vi "UHR-Fleezers Control (fpga) - Leonardo 04-2018 V3.vi"() -> ()   [LabVIEW 2013]
doc: "UHR-Fleezers Instrument Control Code (fpga)"
uses:
  <vilib>/Platform/TimedLoop/XDataNode/timing_clust.ctl
  <vilib>/Platform/TimedLoop/XDataNode/nitl_modes.ctl
  <vilib>/Platform/TimedLoop/XDataNode/wakeup.ctl
  <vilib>/rvi/eio/common/nirviEmuTemplateMethod_errors.vi
  <vilib>/rvi/Emulation/niFpgaSctlEmulationGetInTimedLoop.vi
  <vilib>/rvi/Emulation/niFpgaEmulationReportErrorSimple.vi
  <vilib>/rvi/Emulation/niFpgaGetClockAttributes.vi
  <vilib>/rvi/Emulation/niFpgaCriticalErrorInLSC.vi
  <vilib>/rvi/FIFO/Fifo_Resource/nirvififoEmulationReadFpgaImpl.vi
  <vilib>/rvi/DataTransferAndStorage/Container/Common/niFpgaContainerGetUniqueNameForEmu.vi
  <vilib>/rvi/DataTransferAndStorage/Container/Common/niFpgaContainerExecOnDevCompGetState.vi
  <vilib>/rvi/interface/RandomDataEmulation/nirviRandomDataFPGAFIFO.vi
  <vilib>/rvi/interface/RandomDataEmulation/niFpgaRandomDataHandleErrors.vi
  <vilib>/rvi/eio/common/nirviEmuReportErrorAndStop.vi
  <vilib>/rvi/Emulation/niFpgaProcessEmulError.vi
  <vilib>/rvi/FIFO/Fifo_Resource/nirvififoEmulationWriteFpgaImpl.vi
  <vilib>/Platform/TimedLoop/XDataNode/XDataNode.xnode
  <vilib>/eio/EIOMethodNode/EIOMethodNode.xnode
  <vilib>/eio/EIONode/EIONode.xnode
  <vilib>/rvi/DataTransferAndStorage/Container/XNode/niFpgaContainer.xnode
  <vilib>/rvi/FIFO/Fifo_Resource/nirvififoEmulationRead.vi
  <vilib>/rvi/FIFO/Fifo_Resource/niFpgaFifoEmulationRefIn.vi
  <vilib>/rvi/interface/RandomDataEmulation/nirviRandomDataFpgaReadWriteTemplate.vi
  <vilib>/rvi/FIFO/Fifo_Resource/nirvififoEmulationWrite.vi
  <vilib>/addons/control/pid/fpga.llb/XNode/niFpgaPID.xnode
  <vilib>/Platform/TimedLoop/XDataNode/XDNodeRunTimeDep.lvlib
  <vilib>/rvi/Memory/Memory_Emulation/niFpgaMemoryEmulationRefIn.vi
panel:
  in  "Tab Control 2":T1(tab)
  out "BD1 amplitude 1 out":u16
  out "BD1 amplitude 2 out":u16
  in  "FB output range":cluster{"output low":i16, "output high":i16}={"output low"=0, "output high"=3000}
  in  "FB Gains":T2={"proportional gain (Kc)"=10, "integral gain (Kc*Ts/Ti)"=5, "derivative gain (Kc*Td/Ts)"=0}
  in  "RF synth green feedback max":i16=4000
  in  "RD":bool=TRUE
  in  "Swap F1 and F2":bool
  in  "Scan BD":bool
  in  "Start scan":bool
  in  "OSK Bd 1":bool
  in  "Reset Bd 1":bool
  in  "PMODE":bool=TRUE
  in  "Number Interlace Cycles":u8=2 min=1 max=3
  in  "Interlace Off Parameters":u8=1 min=1 max=3
  in  "Interlace ON/OFF":bool
  out "DIO Relative phase":i16
  in  "Phase count adjustment (DIO)":i16
  in  "+ phase (DIO)":bool
  out "DIO Late Counter":u8
  in  "DIO count 1 (ticks)":u16=400
  in  "DIO count 2 (ticks)":u16=400
  in  "DIO count 3 (ticks)":u16=400
  out "AI2 Y Sum Set 2":i16
  out "AI2 Y Sum Set 1":i16
  in  "FB Setpoint Set 1":i16 min=0 step=1
  in  "FB Reset Set 1":bool
  in  "FB On/Off Set 1":bool
  in  "FB Reset Set 2":bool
  in  "FB On/Off Set 2":bool
  in  "FB Setpoint Set 2":i16 min=0 step=1
  in  "Amp switch delay":u8=5
  in  "RF synth bd controls green":bool
  in  "Phase Trap 2":fxp<+,14,14>
  in  "Phase Trap 1":fxp<+,14,14>
  in  "Phase offset method":u8
  in  "BD 2 Amplitude 1":u16
  in  "BD 1 Amplitude 1":u16
  in  "BD 2 Frequency 1":u64
  in  "BD 1 Frequency 1":u64
  in  "BD 2 Amplitude 2":u16
  in  "BD 1 Amplitude 2":u16
  in  "BD 2 Frequency 2":u64
  in  "BD 1 Frequency 2":u64
  in  "BD 2 Amplitude 3":u16
  in  "BD 1 Amplitude 3":u16
  in  "BD 2 Frequency 3":u64
  in  "BD 1 Frequency 3":u64
  in  "BD 2 Delay (Ticks)":u8 caption="Count(Ticks)"
  in  "Next trap write delay (ticks)":u8 caption="Count(Ticks)"
  out "Random phase generated":fxp<+,14,14>
  in  "RF phase reset before cycles":bool
  in  "Trap 1 osc enable":bool
  in  "N trap osc periods":i16
  in  "Trap osc period (pts)":i16
  in  "Osc traps":bool
  in  "Initiate trap osc":bool
  in  "Ready Write":bool
  in  "Data":i64
  in  "Address 2":u32
  in  "Osc trap cont.":bool
  in  "Trap 2 osc enable":bool
  out "green FB running":bool
  in  "APD 2 AO scale factor":i16=1
  in  "BD 1 Delay (ticks)":u8
  in  "Tab Control":T3(tab)=enum."MCL trap control"
  in  "Set 3":bool
  in  "Set 2":bool=TRUE
  in  "Set 1":bool=TRUE
  in  "Trap Pos to FIFO":bool
  in  "N of AI1 Int Acq Sets":i16=2 min=1 max=3 step=1
  out "AI Late Counter":u8
  in  "ai count":u16=400
  in  "+ phase":bool
  in  "Phase count adjustment":i16
  out "Relative phase":i16
  in  "AI to FIFO":bool
  out "BD1 Frequency Out 1":u64
  out "BD1 Frequency Out 2":u64
  out "Trap Pos FIFO Timeout":u16
  out "Trap AI FIFO Timeout":u16
  in  "Trap FIFO Set Timeout":i32
  in  "Scan freq.  increment":i64
  in  "Scan steps":u64
  in  "Number of scans":u16
  in  "Cycles per step":u64
  in  "Raster setpoint":fxp<+/-,16,1>
  in  "Raster to target force":bool
  out "Actual Scan freq":u64
  in  "Cont. Scan":bool
  out "Scan I":u64
  in  "Abort scan":bool
  out "Scanning":bool
  in  "FB Min frequency":u64
  in  "FB Max Frequency":u64
  in  "Dynamic Force FB (Ronen)":bool
  in  "Trap pos. FB Range":T4={"FB2 output low"=-1.0, "FB2 output high"=0.999969482421875}
  in  "Trap Pos. FB Gains":T5={"proportional gain (Kc)"=0.999969482421875, "integral gain (Kc*Ts/Ti)"=0.999969482421875, "derivative gain (Kc*Td/Ts)"=0.0}
  in  "B factor":fxp<+/-,32,16>
  in  "Negate Diff?":bool
  in  "Diff FB Measurement?":bool
  in  "FB Trig Integrate":u32=1
  out "TTrig?":bool
  in  "TTrig Negate Pos":bool=TRUE
  out "Trap Pos FB Int Signal":fxp<+/-,24,9> format="%.18g"
  out "Trap Pos FB Int-Norm Signal":fxp<+/-,16,1> format="%.16g"
  in  "FPGA TTrig Thresh":i64
  in  "FPGA Trap Trig":bool
  out "Trap Pos FB Action":i64
  in  "Trap Pos. FB Offset Factor":i64
  in  "Trap Pos. FB Mult Factor":i64=2
  in  "Trap Pos. FB Reset":bool
  in  "Trap Pos FB Monitor T1 or T2":bool
  in  "AI1 X Scale":u16
  in  "Trap Pos FB Int Count":u16=100
  in  "Trap Pos FB Negate Action":bool
  out "AI1 X Set 2":fxp<+/-,16,1>
  out "AI1 X Set 1":fxp<+/-,16,1>
  in  "Trap Pos. FB SP":fxp<+/-,16,1>
  in  "Force feedback":bool
  out "TTrig Sig":i64
  out "TTrig Fin Thresh":i64
  in  "1D or 2D Scan?":bool
  in  "Abort scan (MCL)":bool
  in  "MCL Scan Axis":bool
  in  "Cont. Scan (MCL)":bool
  out "Scan I (MCL)":u64
  in  "Number of scans (MCL)":u16
  out "Scanning MCL":bool
  in  "Scan steps (MCL)":u64
  in  "Cycles per step (MCL)":u64
  in  "Scan freq.  increment (MCL)":i16
  in  "Start scan (MCL)":bool
  in  "AO2 (X)":i16
  in  "AO1 (Y)":i16
  out "MCL Late Counter":u8
  in  "MCL count":u32=800
  out "MCL Relative Phase":i16
  in  "Phase count adjustment (MCL)":i16
  in  "+ phase (MCL)":bool
  in  "Lifetime events to read blue":u16=100
  in  "Lifetime read blue fifo":bool
  out "lifetime events in fifo":u16
  in  "APD Gate Operating Mode":u8 max=2 step=1
  in  "Invert APD Gate":bool
  in  "APD Gate OFF Count":u16=100
  in  "APD Gate ON Count":u16=300
  out "APD 1 Gate Late Counter":u8
  out "APD 1 Gate Relative Phase":i16
  in  "Phase count adjustment (APD 1 Gate)":i16
  in  "+ phase (APD 1 Gate)":bool
  out "APD 2 Counts 0":u32
  out "APD 2 Counts 1":u32
  out "APD 1 Counts 0":u32
  out "APD 1 Counts 1":u32
  in  "Lifetime timeout APD1":u16=200
  in  "APD to FIFO":bool
  in  "APD Acq Rate Count":u32=20000000
  out "APD Acq Late Counter":u16
  out "APD Acq Relative Phase":i16
  in  "+ phase (APD Acq)":bool
  in  "Phase Count Adjustment (APD Acq)":i16
  in  "APD 1 AO scale factor":i16=1
  out "APD2 out state":bool
  out "APD1 out state":bool
  out "APD Acq Late?":bool
  in  "D3 2":i16
  in  "I3 2":i16=5
  in  "P3 2":i16=10
  in  "Green FB Setpoint 2":i16=250 min=0 step=1
  in  "Green FB Reset 2":bool
  in  "Green Filter Flipper":bool
  in  "Green interlace OFF count":u16=100
  out "GI Relative phase":i16
  in  "Phase count adjustment (GI)":i16
  in  "+ phase (GI)":bool
  in  "Green interlace ON count":u16=300
  out "GI Late Counter":u8
  in  "Invert GI":bool
  in  "Operating Mode":u8 max=2 step=1
  in  "Current Out":u16=30000
  in  "Green int current ON count adj":u32=150
  in  "Green interlace OFF count 2":u32=900
  in  "Green interlace ON count 2":u32=300
  out "GI Late Counter 2":u16
  in  "Green FB Count":u32=1200
  in  "Phase count adjustment (GI) 2":i16=20
  in  "Green FB Setpoint":i16=250 min=0 step=1
  in  "Invert GI 2":bool
  out "GI Relative phase 2":i16
  in  "+ phase (GI) 2":bool
  in  "Phase count adjustment (Green FB)":i16=10
  out "Green Late Counter":u16
  out "Green FB Relative Phase":i16
  in  "+ phase (Green FB)":bool
  out "Green FB Signals":T6
  out "Green FB Sum":i16
  in  "Green FB Gains":T2={"proportional gain (Kc)"=10, "integral gain (Kc*Ts/Ti)"=5, "derivative gain (Kc*Td/Ts)"=0}
  in  "Green FB On/Off":bool
  in  "Green FB Reset":bool
  out "Green FB Late?":bool
  out "GI Late?":bool
  in  "Operating Mode 2":u8=2 max=2 step=1
  in  "Chassis2/Mod4/AO1":u16
  in  "+ phase (RI)":bool
  out "RI Relative phase":i16
  out "RI Late Counter":u8
  in  "Red interlace ON count":u16=300
  in  "Red interlace OFF count":u16=100
  in  "Invert RI":bool
  in  "Red Laser Operating Mode":u8 max=2 step=1
  in  "Phase count adjustment (RI)":i16
  in  "Phase count adjustment (BI D)":i16
  in  "Blue Laser Operating Mode (D)":u8 max=2 step=1
  in  "Invert BI (D)":bool
  in  "Blue interlace OFF count (D)":u16=100
  in  "Blue interlace ON count (D)":u16=300
  out "Blue Late Counter (D)":u8
  out "BI Relative phase (D)":i16
  in  "+ phase (BI D)":bool
  in  "Lifetime to FIFO":bool
  out "lifetime (ticks)":u16
  # "Raster Scan AOD"
  # "1 (X)"
  # "2 (Y)"
  # "IR Intensity Feedback (RF BD 1)"
  # "FB Gains Set 1"
  # "FB output range 1"
  # "IR Intensity Feedback (RF BD 2) -\nonly when using BD 2 for green laser AOM (not trap Y)"
  # "Keep below 4096 (12 bits) to stay within range of RF board. Going over doesn't saturate, it truncates higher bits."
  # "RF phase offset control"
  # "Methods are:\n0 - Default, do nothing at all (no phase offset writes)\n1 - Manual phase adjustment\n2 - Cycle the phase adjustment using the input phase numbers as increment values for each cycle"
  # "False is usual, True is external loop method"
  # "Parameters if using the external RF switching loop"
  # "Parameters if using the usual internal RF switching method"
  # "FB Triggering Excitation Laser"
  # "Trap Pos. FB Gains"
  # "Trap Pos. FB Range"
  # "AO1 (Y)"
  # "2D"
  # "Trap 3"
  # "1D"
  # "AO2 (X)"
  # "Fl Laser"
  # "APD AO for aligning"
  # "Detection Loop"
  # "Green fluorescent laser digital gate interlacing loop"
  # "0 Forced ON\n1 Forced OFF\n2 Interlacing"
  # "ALEX settings:"
  # "Controls for usual IA ME controls green AOM"
  # "Controls for RF synth board controls green AOM"
  # "Green FB Gains"
  # "Red fluorescent laser digital gate interlacing loop"
  # "Detection Loop"
  # "0 Forced ON\n1 Forced OFF\n2 Interlacing"
  # "Analog/FB Control Loop\n(Disabled)"
  # "Digital Control Loop"
  # "Blue laser intensity reading"
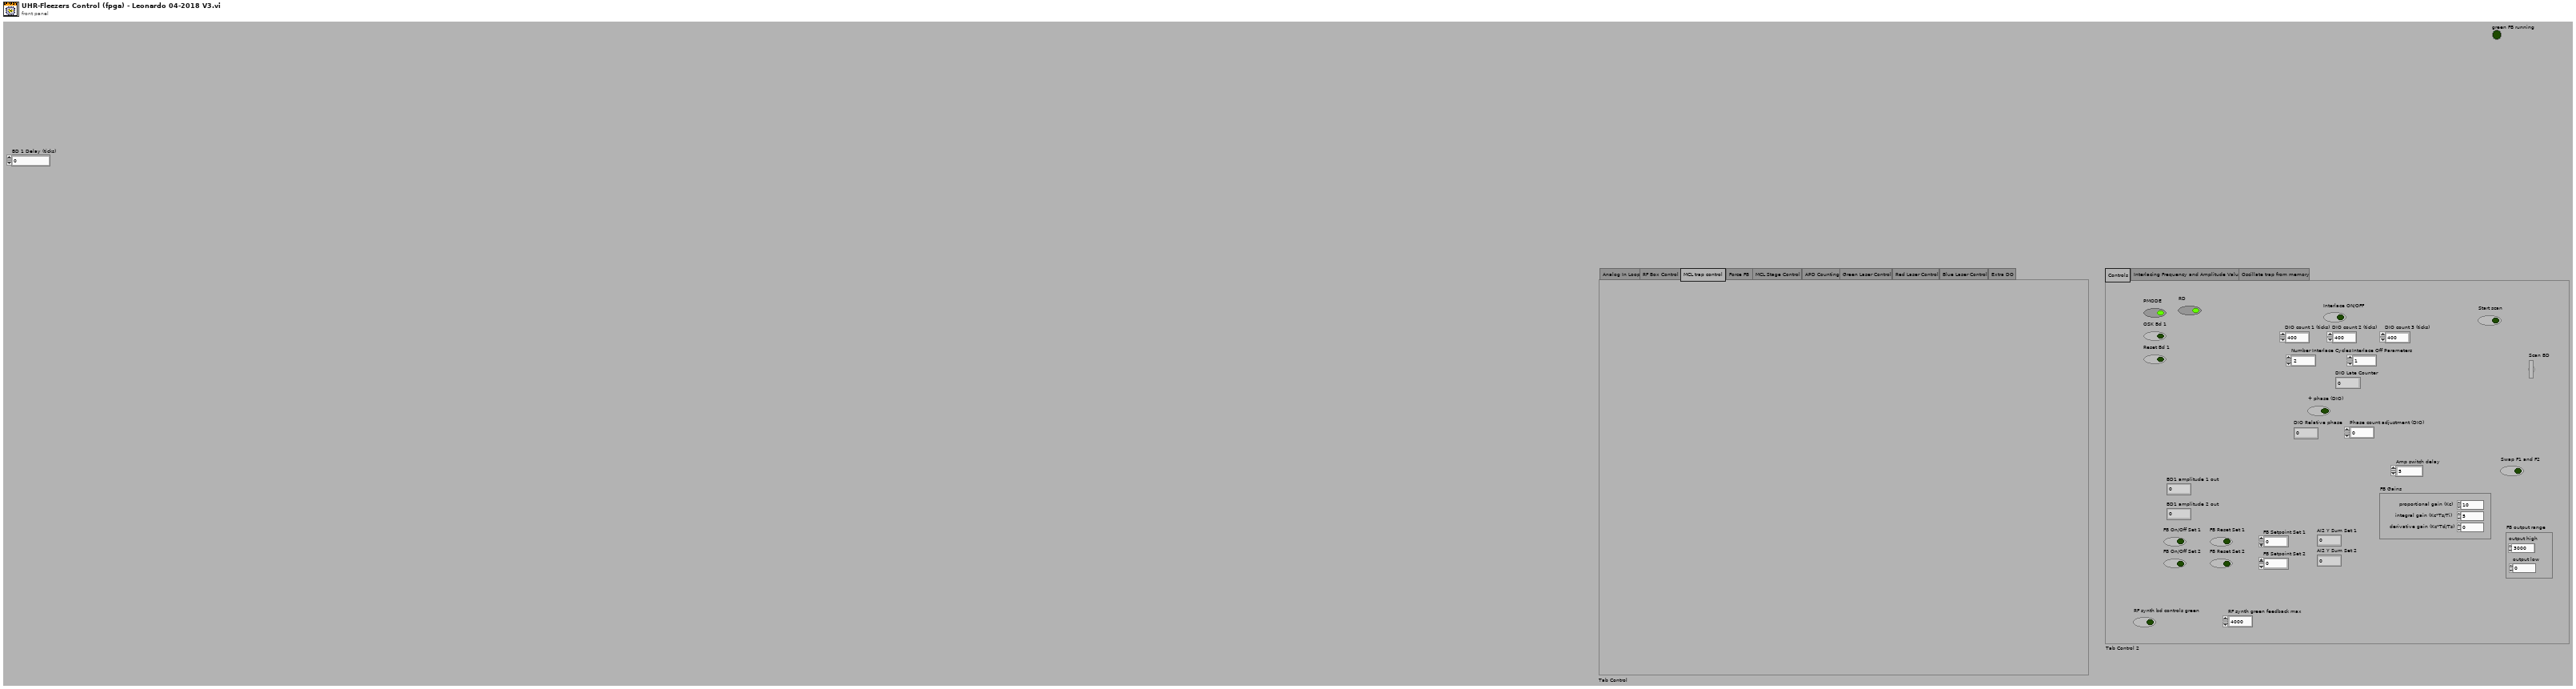
[diagram p1: front panel]
types:
  T1 = enum32{"Controls", "Interlacing Frequency and Amplitude Values", "Oscillate trap from memory"}
  T2 = cluster{"proportional gain (Kc)":i16, "integral gain (Kc*Ts/Ti)":i16, "derivative gain (Kc*Td/Ts)":i16}
  T3 = enum32{"Analog In Loop", "RF Box Control", "MCL trap control", "Force FB", "MCL Stage Control", "APD Counting", "Green Laser Control", "Red Laser Control", "Blue Laser Control", "Extra DO"}
  T4 = cluster{"FB2 output low":fxp<+/-,16,1>, "FB2 output high":fxp<+/-,16,1>}
  T5 = cluster{"proportional gain (Kc)":fxp<+/-,16,1>, "integral gain (Kc*Ts/Ti)":fxp<+/-,16,1>, "derivative gain (Kc*Td/Ts)":fxp<+/-,16,1>}
  T6 = cluster{"Green FB Ch 0":i16, "Green FB Ch 1":i16, "Green FB Ch 2":i16}
  T7 = typedef "XDNodeRunTimeDep.lvlib/timing_clust.ctl" = cluster{"Expected End [f-1]":u64, "Actual End [f-1]":u64, "Finished Late? [f-1]":bool, "Expected End [i-1]":u64, "Actual End [i-1]":u64, "Finished Late? [i-1]":bool, "Expected Start [i]":u64, "Actual Start [i]":u64, "Expected Start [f]":u64, "Actual Start [f]":u64, "Source Name":string, "Structure Name":string, "Period":i64, "Deadline":i64, "Offset":i64, "Start":i64, "Priority":i32, "Timeout":i32, "Mode":T8, "Wakeup Reason":T9, "Error":errorcluster, "Source Type":string, "Secondary Source Type":string, "Global End Time":u64, "Global Start Time":u64, "Frame Duration":u64, "Iteration Duration":u64, "Assigned CPU":i32, "I/O Scan Engine Mode":u32}
  T8 = typedef "XDNodeRunTimeDep.lvlib/nitl_modes.ctl" = enum32{"No Change", "Process missed periods, maintain original phase", "Discard missed periods, maintain original phase", "Process missed periods, ignore original phase", "Discard missed periods, ignore original phase"}
  T9 = typedef "XDNodeRunTimeDep.lvlib/wakeup.ctl" = enum32{"Normal", "Aborted", "Asynchronous wakeup", "Timing source error", "Timed loop error", "Timeout"}
  T10 = cluster{"Chassis2/Mod2/AI0":i16, "Chassis2/Mod2/AI1":i16, "Chassis2/Mod2/AI2":i16}
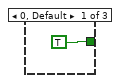
[diagram p3: hidden frame]
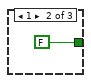
[diagram p4: hidden frame]
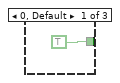
[diagram p8: hidden frame]
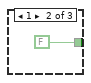
[diagram p9: hidden frame]
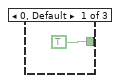
[diagram p10: hidden frame]
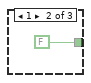
[diagram p11: hidden frame]
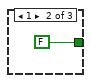
[diagram p13: hidden frame]
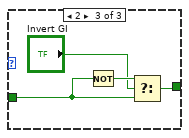
[diagram p14: hidden frame]
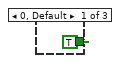
[diagram p15: hidden frame]
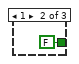
[diagram p16: hidden frame]
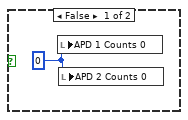
[diagram p17: hidden frame]
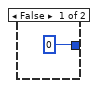
[diagram p19: hidden frame]
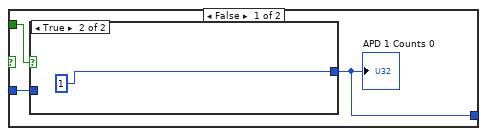
[diagram p20: hidden frame]
diagram:
  w5 = FALSE
  # "BD2 amp"
  # "BD1 amp"
  # "BD2 amp"
  # "BD1 amp"
  # "timing array current index"
  # "timing array"
  # "timing counter (phase adjusted here)"
  # "late counter"
  n1 = while {
    stop <- FALSE stop-if-true
    n2 = xnode "FPGA I/O Node"("Connector0/DIO3"="Green Filter Flipper", "Chassis2/Mod1/AO1"="Chassis2/Mod4/AO1") -> ()  [unwired: 2 in, 2 out]
    n3 = call "Loop Timer11"("Count(Ticks)"=u32 40000 ("Extra DO Counts")) -> ()  [unwired: 1 out]
  }
  n4 = disable-structure shown="Disabled" {
    frame Disabled {
      w20 = i16 2 items=["UnSet Ready", "ReadWrite", "Wait Ready"]
      n5 = while "Handshake memory transfer for trap oscillation sin wave data" {
        shift-right: [w22] -> _
        shift-left: w20 -> [w23]
        stop <- FALSE stop-if-true
        # "Write"
        n6 = case shown="1" w23 {
          tunnel: [w26 w31 w32] -> w22
          frame 3, Default {
            w24 = i16 2 items=["UnSet Ready", "ReadWrite", "Wait Ready"]
            w25 = i16 1 items=["UnSet Ready", "ReadWrite", "Wait Ready"]
            n7 = Select(t=w25, s="Ready Write", f=w24) -> (s? t:f=w26:i16)
          }
          frame 1 {
            w31 = i16 0 items=["UnSet Ready", "ReadWrite", "Wait Ready"]
            n8 = xnode ("Memory Write")("Address"="Address 2", "Data"="Data", "Memory In"=refnum<k21> "Trap osc memory") -> ()  [unwired: 1 out]
          }
          frame 0 {
            w32 = i16 2 items=["UnSet Ready", "ReadWrite", "Wait Ready"]
            n9 = local write "Ready Write"(FALSE ("Ready Read")) -> ()
          }
        }
      }
    }
    frame Enabled {
    }
  }
  n10 = flat-sequence "FPGA initialization to do before running any of the loops" {
    tunnel: [u16 0 ("DIO count 3 (ticks)")] -> w2
    tunnel: [w41] -> _
    frame #0 {
      # "UDCLK out enable and set low"
      # "WR"
      # "BD 2"
      # "BD 1"
      # "With the RF synth board initialization now done in a separate fpga vi, now when this vi is started, board is already configured and is ready for interlacing. Just need to set WR high and enabled UDCLK as write and set to low.\nbefore setting data and address bits."
      # "Start up expansion chassis early\nto avoid delays later"
      # "Set data and address values to something safe (a correct setting) so any initial WR and udclk flipping doesn't have a chance to mess anything up. Safe would be setting an unused data entry:"
      n11 = xnode "FPGA I/O Method Node"("Enable"=TRUE) -> ("FPGA I/O Out"=w35:refnum<k21>)  [unwired: 1 in]
      n12 = xnode "FPGA I/O Method Node"("Enable"=TRUE) -> ("FPGA I/O Out"=w38:refnum<k21>)  [unwired: 1 in]
      n13 = xnode "FPGA I/O Node"("Chassis2/Mod1/AO0"=u16 0 ("Chassis2/Mod4/AO0")) -> ("Chassis2/Mod2/AI0"=w41:i16)  [unwired: 2 in, 2 out]
      n14 = xnode "FPGA I/O Node"("Connector1/DIO15"=TRUE) -> ()  [unwired: 1 in, 1 out]
      n15 = xnode "FPGA I/O Node"("I/O Item"=FALSE ("Connector1/DIO30"), "FPGA I/O In"=w35) -> ()  [unwired: 1 out]
      n16 = xnode "FPGA I/O Node"("I/O Item"=FALSE ("Connector1/DIO30"), "FPGA I/O In"=w38) -> ()  [unwired: 1 out]
      n17 = xnode "FPGA I/O Node"("Connector1/DIO0"=FALSE, "Connector1/DIO1"=FALSE, "Connector1/DIO2"=FALSE, "Connector1/DIO3"=FALSE, "Connector1/DIO4"=FALSE, "Connector1/DIO5"=FALSE, "Connector1/DIO6"=FALSE, "Connector1/DIO7"=FALSE, "Connector1/DIO8"=FALSE, "Connector1/DIO9"=FALSE, "Connector1/DIO10"=FALSE, "Connector1/DIO11"=FALSE, "Connector1/DIO12"=FALSE, "Connector1/DIO13"=FALSE, "Connector1/DIO20"=FALSE, "Connector1/DIO21"=FALSE, "Connector1/DIO22"=FALSE, "Connector1/DIO23"=FALSE, "Connector1/DIO24"=FALSE, "Connector1/DIO25"=FALSE, "Connector1/DIO26"=FALSE, "Connector1/DIO27"=FALSE, "Connector1/DIO14"=FALSE) -> ()  [unwired: 23 in, 23 out]
    }
  }
  n18 = node-c288() -> (w12:T7)  [unwired: 1 in]
  n19 = timed-loop "RF box board DIO control: control bits" {
    timing: w12 -> [_]
    timing-out: [_] -> w11
    tunnel: [w68] -> _
    tunnel: w2 -> [w68]
    stop <- FALSE stop-if-true
    n20 = xnode "FPGA I/O Node"("Connector1/DIO16"="RD", "Connector1/DIO17"="PMODE", "Connector1/DIO18"="OSK Bd 1", "Connector1/DIO19"="Reset Bd 1") -> ()  [unwired: 4 in, 4 out]
  }
  n21 = node-c288(w11) -> ()
  n22 = To Unsigned Long Integer(number=w2) -> (unsigned 32bit integer=w1:u32)
  n23 = To Unsigned Long Integer(number=w2) -> (unsigned 32bit integer=w3:u32)
  n24 = local read "AO1 (Y)"() -> (w14:i16)
  n25 = local read "AO2 (X)"() -> (w13:i16)
  n26 = To Unsigned Long Integer(number=w2) -> (unsigned 32bit integer=w7:u32)
  n27 = while "DAQ AI set 1" {
    shift-right: [w75] -> _
    shift-left: w2 -> [w80]
    stop <- FALSE stop-if-true
    n28 = flat-sequence {
      tunnel: w80 -> [w91]
      tunnel: [w90] -> w78
      tunnel: [w91] -> w77
      tunnel: [w101] -> w88
      tunnel: [w100] -> w87
      tunnel: [w99] -> w86
      tunnel: [w98] -> w85
      tunnel: [w97] -> w84
      tunnel: [w96] -> w83
      tunnel: [w95] -> w82
      tunnel: [w94] -> w81
      tunnel: [w93] -> w79
      tunnel: w78 -> [w93]
      tunnel: w77 -> [w92]
      tunnel: [w92] -> w76
      tunnel: [w131] -> w75
      tunnel: w88 -> [w157]
      tunnel: w87 -> [w123]
      tunnel: w86 -> [w124]
      tunnel: w85 -> [w103]
      tunnel: w84 -> [w147]
      tunnel: w83 -> [w146]
      tunnel: w82 -> [w145]
      tunnel: w81 -> [w144]
      tunnel: w79 -> [w141]
      tunnel: w76 -> [w138]
      frame #0 {
        n29 = call "Loop Timer"("Count(Ticks)"=w91) -> ("Tick Count(Ticks)"=w90:u32)
      }
      frame #1 {
        n30 = xnode "FPGA I/O Node"("Connector1/DIO31"=TRUE ("Connector1/DIO33")) -> ("Connector0/AI0"=w101:i16, "Connector0/AI1"=w100:i16, "Connector0/AI2"=w99:i16, "Connector0/AI3"=w98:i16, "Connector0/AI4"=w97:i16, "Connector0/AI5"=w96:i16, "Connector0/AI6"=w95:i16, "Connector0/AI7"=w94:i16)  [unwired: 9 in, 9 out]
      }
      frame #2 {
        w127 = FALSE ("AI to FIFO")
        # "Normalize by trap bead QPD sum, AI3"
        # "Adjust phase after data acquired if button pressed"
        n31 = feedback #1(i16 1) -> (w150:i16)
        n32 = Increment(x=w150) -> (x+1=w156:i16)
        n33 = Scale By Power Of 2(n="AI1 X Scale", x=w123) -> (x*2^n=w121:i16)
        n34 = Greater?(x=w156, y="N of AI1 Int Acq Sets") -> (0:w153:bool)
        n35 = Select(t=i16 1, s=w153, f=w156) -> (s? t:f=w155:i16)
        n36 = feedback-in #1(w155) -> ()
        n37 = Divide(x=w121, y=w103) -> (x/y=w120:fxp<+/-,16,1>)
        n38 = feedback #2(w127) -> (w125:bool)
        n39 = feedback #3(w127) -> (w143:bool)
        n40 = case shown="1, Default" w150 {
          tunnel: w124 -> [w180 w187 _]
          tunnel: ["Set 1" "Set 2" "Set 3"] -> w148
          tunnel: ["AI to FIFO" w189 w194] -> w142
          tunnel: w143 -> [_ w189 w194]
          tunnel: ["Trap Pos to FIFO" w188 w193] -> w126
          tunnel: w125 -> [_ w188 w193]
          tunnel: w120 -> [w179 w186 _]
          tunnel: [w178 w184 FALSE] -> w107
          tunnel: [w177 w185 u64 0 ("BD1 Frequency Out 2")] -> w106
          frame 1, Default {
            n41 = local read "BD1 Frequency Out 1"() -> (w177:u64)
            n42 = Compound Arithmetic op=AND("Trap Pos to FIFO", "Set 1", "AI to FIFO") -> (w178:bool)
            "AI2 Y Sum Set 1" <- w180
            "AI1 X Set 1" <- w179
          }
          frame 2 {
            n43 = local read "BD1 Frequency Out 2"() -> (w185:u64)
            n44 = Compound Arithmetic op=AND(w188, "Set 2", w189) -> (w184:bool)
            "AI2 Y Sum Set 2" <- w187
            "AI1 X Set 2" <- w186
          }
          frame 3 {
          }
        }
        n45 = And(x=w148, y=w142) -> (x .and. y?=w149:bool)
        n46 = case shown="True" w149 {
          tunnel: w157 -> [_ w208]
          tunnel: w123 -> [_ w207]
          tunnel: w124 -> [_ w206]
          tunnel: w103 -> [_ w205]
          tunnel: w147 -> [_ w204]
          tunnel: w146 -> [_ w203]
          tunnel: w145 -> [_ w202]
          tunnel: w144 -> [_ w201]
          tunnel: 0 ("DMA buffer timeout") -> [_ w210]
          frame False {
          }
          frame True {
            n47 = Build Array(w208, w207, w206, w205, w204, w203, w202, w201) -> (w209:i16[])
            n48 = for {
              tunnel: w209 -> [w212] mode=indexing
              tunnel: w210 -> [w213]
              tunnel: [w211] -> w199 mode=indexing
              n49 = xnode ("FIFO Write")("Element"=w212, "Timeout"=w213) -> ("Timed Out?"=w211:bool)  [unwired: 1 in, 1 out]
            }
            n50 = Or Array Elements(Boolean array=w199) -> (logical OR=w196:bool)
            n51 = Boolean To (0,1)(Boolean=w196) -> (0, 1=w198:i16)
            n52 = feedback #4(u16 0) -> (w197:u16)
            n53 = Add(x=w198, y=w197) -> (x+y=w195:u16)
            "Trap AI FIFO Timeout" <- w195
            n54 = feedback-in #4(w195) -> ()
          }
        }
        n55 = feedback-in #2(w126) -> ()
        n56 = feedback-in #3(w142) -> ()
        n57 = case shown="True" w107 {
          tunnel: w106 -> [_ w163]
          tunnel: [u8 0 w160] -> w105
          frame False {
          }
          frame True {
            n58 = Split Number(x=w163) -> (hi(x)=w164:u32, lo(x)=w165:u32)
            n59 = Split Number(x=w164) -> (lo(x)=w166:u16)  [unwired: 1 out]
            n60 = Split Number(x=w165) -> (hi(x)=w167:u16, lo(x)=w168:u16)
            n61 = Build Array "BD 1 nu Stack"(w166, w167, w168) -> (w162:u16[])
            n62 = for {
              tunnel: w162 -> [w175] mode=indexing
              shift-right: [w171] -> w160
              shift-left: u8 0 -> [w172]
              n63 = xnode ("FIFO Method Node")("Element"=w175, "Timeout"="Trap FIFO Set Timeout") -> ("Timed Out?"=w174:bool)  [unwired: 1 in, 1 out]
              n64 = Boolean To (0,1)(Boolean=w174) -> (0, 1=w173:i16)
              n65 = To Unsigned Byte Integer(number=w173) -> (unsigned 8bit integer=w170:u8)
              n66 = Add(x=w170, y=w172) -> (x+y=w171:u8)
            }
          }
        }
        n67 = To Unsigned Word Integer(number=w105) -> (unsigned 16bit integer=w104:u16)
        n68 = feedback #5(u16 0) -> (w118:u16)
        n69 = Add(x=w104, y=w118) -> (x+y=w117:u16)
        "Trap Pos FIFO Timeout" <- w117
        n70 = feedback-in #5(w117) -> ()
        n71 = feedback-in #6(w141) -> ()
        n72 = feedback #6(w141) -> (w140:u32)
        n73 = Subtract(x=w141, y=w140) -> (x-y=w139:u32)
        n74 = xnode "FPGA I/O Node"("Connector1/DIO31"=FALSE ("Connector1/DIO34")) -> ()  [unwired: 1 in, 1 out]
        n75 = Subtract(x=w139, y=w138) -> (x-y=w109:u32)
        n76 = Boolean To (0,1)(Boolean="+ phase") -> (0, 1=w134:i16)
        n77 = Multiply(x=w134, y="Phase count adjustment") -> (x*y=w128:i16)
        n78 = Subtract(x="ai count", y=w109) -> (x-y=w132:u32)
        n79 = Number To Boolean Array(number=w109) -> (Boolean array=w110:bool[])
        n80 = feedback #7(i16 0) -> (w130:i16)
        n81 = Add(x=w132, y=w128) -> (x+y=w131:u32)
        n82 = Subtract(x=w130, y=w128) -> (x-y=w129:i16)
        "Relative phase" <- w129
        n83 = feedback-in #7(w129) -> ()
        n84 = Or Array Elements(Boolean array=w110) -> (logical OR=w108:bool)
        n85 = Boolean To (0,1)(Boolean=w108) -> (0, 1=w115:i16)
        n86 = To Unsigned Byte Integer(number=w115) -> (unsigned 8bit integer=w112:u8)
        n87 = feedback #8(u8 0) -> (w113:u8)
        n88 = Add(x=w112, y=w113) -> (x+y=w111:u8)
        "AI Late Counter" <- w111
        n89 = feedback-in #8(w111) -> ()
      }
    }
  }
  n90 = while "MCL stage control" {
    shift-right: [w226] -> _
    shift-left: w2 -> [w229]
    shift-right: [w219] -> _
    shift-left: w14 -> [w216]
    shift-right: [w218] -> _
    shift-left: w13 -> [w214]
    stop <- FALSE stop-if-true
    n91 = flat-sequence {
      tunnel: w229 -> [w232]
      tunnel: [w231] -> w225
      tunnel: [w232] -> w223
      tunnel: [w234] -> w217
      tunnel: w216 -> [w234]
      tunnel: [w233] -> w215
      tunnel: w214 -> [w233]
      tunnel: w225 -> [w238]
      tunnel: [w238] -> w224
      tunnel: w223 -> [w237]
      tunnel: [w237] -> w222
      tunnel: w217 -> [w236]
      tunnel: w215 -> [w235]
      tunnel: w224 -> [w246]
      tunnel: w222 -> [w245]
      tunnel: [w246] -> w228
      tunnel: [w245] -> w227
      tunnel: [w244] -> w221
      tunnel: [w243] -> w220
      tunnel: [w318] -> w226
      tunnel: w228 -> [w325]
      tunnel: w227 -> [w322]
      tunnel: w221 -> [w320]
      tunnel: w220 -> [w319]
      tunnel: [w320] -> w219
      tunnel: [w319] -> w218
      frame #0 {
        n92 = call "Loop Timer3"("Count(Ticks)"=w232) -> ("Tick Count(Ticks)"=w231:u32)
      }
      frame #1 {
        n93 = xnode "FPGA I/O Node"("Connector0/AO1"=w236, "Connector0/AO2"=w235) -> ()  [unwired: 2 in, 2 out]
      }
      frame #2 {
        n94 = local read "Scanning MCL"() -> (w258:bool)
        n95 = Or(x=w258, y="Start scan (MCL)") -> (x .or. y?=w253:bool)
        n96 = Not(x="Abort scan (MCL)") -> (.not. x?=w251:bool)
        n97 = And(x=w251, y=w253) -> (x .and. y?=w250:bool)
        n98 = case "Raster scan" shown="False" w250 {
          tunnel: [w259 w302] -> w255
          tunnel: "Start scan (MCL)" -> [_ w287]
          tunnel: [w259 w263] -> w239
          frame False {
            w259 = i16 0
            n99 = local write "Scanning MCL"(FALSE ("scanning")) -> ()
          }
          frame True {
            w273 = i16 0
            w272 = u64 0
            # "scan incr."
            # "freq. incr. mult."
            # "count steps"
            # "count number of cycles"
            n100 = feedback #9(w272) -> (w299:u64)
            n101 = Select(t=w272, s=w287, f=w299) -> (s? t:f=w301:u64)
            n102 = Increment(x=w301) -> (x+1=w298:u64)
            n103 = Greater?(x="Cycles per step (MCL)", y=w298) -> (0:w282:bool)
            n104 = Select(t=w298, s=w282, f=w272) -> (s? t:f=w297:u64)
            n105 = feedback-in #9(w297) -> ()
            n106 = feedback #10(w272) -> (w296:u64)
            n107 = Select(t=w272, s=w287, f=w296) -> (s? t:f=w291:u64)
            n108 = Increment(x=w291) -> (x+1=w295:u64)
            n109 = Add(x="Scan steps (MCL)", y="Scan steps (MCL)") -> (x+y=w294:u64)
            n110 = Select(t=w291, s=w282, f=w295) -> (s? t:f=w277:u64)
            n111 = Greater?(x=w294, y=w277) -> (0:w276:bool)
            n112 = Select(t=w277, s=w276, f=w272) -> (s? t:f=w292:u64)
            n113 = feedback-in #10(w292) -> ()
            n114 = Equal?(x="Scan steps (MCL)", y=w277) -> (x = y?=w281:bool)
            n115 = Greater?(x="Scan steps (MCL)", y=w291) -> (0:w290:bool)
            n116 = feedback #11(w273) -> (w293:i16)
            n117 = Select(t=w273, s=w287, f=w293) -> (s? t:f=w279:i16)
            n118 = Increment(x=w279) -> (x+1=w289:i16)
            n119 = Decrement(x=w279) -> (x-1=w288:i16)
            n120 = Select(t=w289, s=w290, f=w288) -> (s? t:f=w280:i16)
            n121 = Select(t=w279, s=w281, f=w280) -> (s? t:f=w278:i16)
            n122 = Select(t=w279, s=w282, f=w278) -> (s? t:f=w274:i16)
            n123 = Select(t=w274, s=w276, f=w273) -> (s? t:f=w275:i16)
            n124 = feedback-in #11(w275) -> ()
            n125 = feedback #12(w272) -> (w286:u64)
            n126 = Select(t=w272, s=w287, f=w286) -> (s? t:f=w261:u64)
            n127 = Increment(x=w261) -> (x+1=w283:u64)
            n128 = Select(t=w261, s=w276, f=w283) -> (s? t:f=w262:u64)
            n129 = Greater?(x="Number of scans (MCL)", y=w262) -> (0:w269:bool)
            n130 = Multiply(x="Scan freq.  increment (MCL)", y=w279) -> (x*y=w302:i16)
            n131 = Select(t=TRUE, s="Cont. Scan (MCL)", f=w269) -> (s? t:f=w268:bool)
            "Scanning MCL" <- w268
            n132 = Select(t=w262, s=w268, f=w272) -> (s? t:f=w284:u64)
            n133 = feedback-in #12(w284) -> ()
            n134 = Increment(x=w262) -> (x+1=→"Scan I (MCL)":u64)
            n135 = To Word Integer(number=w261) -> (16bit integer=w264:i16)
            n136 = Multiply(x=w264, y="Scan freq.  increment (MCL)") -> (x*y=w263:i16)
          }
        }
        n137 = Select(t=w239, s="1D or 2D Scan?", f=i16 0) -> (s? t:f=w240:i16)
        n138 = Select(t=w255, s="MCL Scan Axis", f=w240) -> (s? t:f=w256:i16)
        n139 = Select(t=w240, s="MCL Scan Axis", f=w255) -> (s? t:f=w254:i16)
        n140 = Add(x="AO2 (X)", y=w254) -> (x+y=w243:i16)
        n141 = Add(x="AO1 (Y)", y=w256) -> (x+y=w244:i16)
      }
      frame #3 {
        n142 = feedback-in #13(w325) -> ()
        n143 = feedback #13(w325) -> (w324:u32)
        n144 = Boolean To (0,1)(Boolean="+ phase (MCL)") -> (0, 1=w316:i16)
        n145 = Subtract(x=w325, y=w324) -> (x-y=w323:u32)
        n146 = Multiply(x=w316, y="Phase count adjustment (MCL)") -> (x*y=w312:i16)
        n147 = Subtract(x=w323, y=w322) -> (x-y=w304:u32)
        n148 = Subtract(x="MCL count", y=w304) -> (x-y=w314:u32)
        n149 = feedback #14(i16 0) -> (w313:i16)
        n150 = Subtract(x=w313, y=w312) -> (x-y=w311:i16)
        "MCL Relative Phase" <- w311
        n151 = feedback-in #14(w311) -> ()
        n152 = Number To Boolean Array(number=w304) -> (Boolean array=w305:bool[])
        n153 = Or Array Elements(Boolean array=w305) -> (logical OR=w303:bool)
        n154 = Boolean To (0,1)(Boolean=w303) -> (0, 1=w310:i16)
        n155 = Add(x=w314, y=w312) -> (x+y=w318:u32)
        n156 = To Unsigned Byte Integer(number=w310) -> (unsigned 8bit integer=w307:u8)
        n157 = feedback #15(u8 0) -> (w308:u8)
        n158 = Add(x=w307, y=w308) -> (x+y=w306:u8)
        "MCL Late Counter" <- w306
        n159 = feedback-in #15(w306) -> ()
      }
    }
  }
  n160 = while "APD 2 Counter" {
    shift-right: [w329] -> _
    shift-left: w1 -> [w330]
    shift-right: [w328] -> _
    shift-left: _ -> [w327]
    stop <- FALSE stop-if-true
    n161 = flat-sequence {
      tunnel: w330 -> [w338]
      tunnel: [w337] -> w329
      tunnel: [w334] -> w328
      tunnel: w327 -> [w336]
      frame #0 {
        n162 = xnode "FPGA I/O Method Node"("FPGA I/O In"=refnum<k21> "Connector0/DIO1" ("APD 2 DO"), "Timeout"=-1) -> ()  [unwired: 2 out]
      }
      frame #1 {
        n163 = xnode "FPGA I/O Node"() -> ("Connector0/DIO9"=w335:bool, "Connector0/DIO6"=w334:bool)  [unwired: 2 in, 2 out]
        n164 = case shown="True" w335 {
          tunnel: w338 -> [_ w341]
          tunnel: [u32 0 w340] -> w337
          tunnel: w334 -> [_ w343]
          tunnel: w336 -> [_ w342]
          frame False {
          }
          frame True {
            n165 = case shown="True" w343 {
              tunnel: w342 -> [w346 w351]
              tunnel: w341 -> [w345 w352]
              tunnel: [w344 w350] -> w340
              frame False {
                n166 = case shown="True" w346 {
                  tunnel: w345 -> [w348 _]
                  tunnel: [w347 u32 1] -> w344
                  frame False {
                    n167 = Increment(x=w348) -> (x+1=w347:u32)
                  }
                  frame True {
                  }
                }
                "APD 2 Counts 0" <- w344
              }
              frame True {
                n168 = case shown="True" w351 {
                  tunnel: w352 -> [_ w355]
                  tunnel: [u32 1 w354] -> w350
                  frame False {
                  }
                  frame True {
                    n169 = Increment(x=w355) -> (x+1=w354:u32)
                  }
                }
                "APD 2 Counts 1" <- w350
              }
            }
          }
        }
      }
    }
  }
  n170 = while "Green fluorescent laser interlacing (Current to IA 532 nm AOM ME amp)." {
    shift-right: [w361] -> _
    shift-left: w2 -> [w364]
    shift-right: [w358] -> _
    shift-left: i16 0 -> [w356]
    stop <- FALSE stop-if-true
    n171 = flat-sequence {
      tunnel: w364 -> [w367]
      tunnel: [w368] -> w363
      tunnel: [w367] -> w362
      tunnel: [w366] -> w357
      tunnel: w356 -> [w366]
      tunnel: [w371] -> w360
      tunnel: w363 -> [w371]
      tunnel: [w370] -> w359
      tunnel: w362 -> [w370]
      tunnel: w357 -> [w369]
      tunnel: [w384] -> w361
      tunnel: [w400] -> w358
      tunnel: w360 -> [w413]
      tunnel: w359 -> [w410]
      frame #0 {
        n172 = call "Loop Timer10"("Count(Ticks)"=w367) -> ("Tick Count(Ticks)"=w368:u32)
      }
      frame #1 {
        n173 = xnode "FPGA I/O Node"("Chassis2/Mod1/AO0"=w369) -> ()  [unwired: 1 in, 1 out]
      }
      frame #2 {
        n174 = local read "RF synth bd controls green"() -> (w375:bool)
        n175 = Subtract(x="Green interlace OFF count 2", y="Green int current ON count adj") -> (x-y=w393:u32)
        n176 = feedback-in #16(w413) -> ()
        n177 = feedback #16(w413) -> (w412:u32)
        n178 = Add(x="Green int current ON count adj", y="Green interlace ON count 2") -> (x+y=w394:u32)
        n179 = Subtract(x=w413, y=w412) -> (x-y=w411:u32)
        n180 = Subtract(x=w411, y=w410) -> (x-y=w377:u32)
        n181 = Not(x=w375) -> (.not. x?=w373:bool)
        n182 = Number To Boolean Array(number=w377) -> (Boolean array=w378:bool[])
        n183 = Boolean To (0,1)(Boolean="+ phase (GI) 2") -> (0, 1=w390:i16)
        n184 = Or Array Elements(Boolean array=w378) -> (logical OR=w376:bool)
        "GI Late?" <- w376
        n185 = Boolean To (0,1)(Boolean=w376) -> (0, 1=w383:i16)
        n186 = Multiply(x=w390, y="Phase count adjustment (GI) 2") -> (x*y=w386:i16)
        n187 = To Unsigned Word Integer(number=w383) -> (unsigned 16bit integer=w379:u16)
        n188 = feedback #17(u16 0) -> (w381:u16)
        n189 = Add(x=w379, y=w381) -> (x+y=w380:u16)
        "GI Late Counter 2" <- w380
        n190 = feedback-in #17(w380) -> ()
        n191 = feedback #18(i16 0) -> (w387:i16)
        n192 = Subtract(x=w387, y=w386) -> (x-y=w385:i16)
        "GI Relative phase 2" <- w385
        n193 = feedback-in #18(w385) -> ()
        n194 = feedback #19(TRUE) -> (w405:bool)
        n195 = case shown="2" "Operating Mode 2" {
          tunnel: [TRUE FALSE w430] -> w395
          tunnel: w405 -> [_ _ w427]
          frame 0, Default {
          }
          frame 1 {
          }
          frame 2 {
            n196 = Not(x=w427) -> (.not. x?=w429:bool)
            n197 = Select(t=w429, s="Invert GI 2", f=w427) -> (s? t:f=w430:bool)
          }
        }
        n198 = And(x=w395, y="Green FB On/Off") -> (x .and. y?=w374:bool)
        "green FB running" <- w374
        n199 = And(x=w374, y=w373) -> (x .and. y?=w372:bool)
        n200 = case shown="True" w372 {
          tunnel: "Current Out" -> [w414 _]
          tunnel: [w414 w419] -> w399
          frame False {
          }
          frame True {
            n201 = local read "Green FB Sum"() -> (w415:i16)
            n202 = call "Slower PID.vi"("process variable"=w415, "reset?"="Green FB Reset", "setpoint"="Green FB Setpoint", "PID gains (x 2^8)"="Green FB Gains", "output range"=cluster{"output high":i16, "output low":i16} {"output high"=32767, "output low"=-32768} ("Green FB output range")) -> ("output"=w423:i16)  [unwired: 10 out]
            n203 = To Long Integer(number=w423) -> (32bit integer=w416:i32)
            n204 = Add(x=w416, y=32768) -> (x+y=w418:i32)
            n205 = To Unsigned Word Integer(number=w418) -> (unsigned 16bit integer=w419:u16)
          }
        }
        n206 = Not(x=w405) -> (.not. x?=w402:bool)
        n207 = Select(t=w394, s=w402, f=w393) -> (s? t:f=w407:u32)
        n208 = Subtract(x=w407, y=w377) -> (x-y=w388:u32)
        n209 = Add(x=w388, y=w386) -> (x+y=w384:u32)
        n210 = feedback-in #19(w402) -> ()
        n211 = Boolean To (0,1)(Boolean=w395) -> (0, 1=w401:i16)
        n212 = To Unsigned Word Integer(number=w401) -> (unsigned 16bit integer=w398:u16)
        n213 = Multiply(x=w398, y=w399) -> (x*y=w400:u16)
      }
    }
  }
  n214 = while "APD 1 Counter" {
    shift-right: [w432] -> _
    shift-left: w3 -> [w434]
    shift-right: [w433] -> _
    shift-left: _ -> [w431]
    stop <- FALSE stop-if-true
    n215 = flat-sequence {
      tunnel: w434 -> [w442]
      tunnel: [w439] -> w433
      tunnel: [w441] -> w432
      tunnel: w431 -> [w438]
      frame #0 {
        n216 = xnode "FPGA I/O Method Node"("FPGA I/O In"=refnum<k21> "Connector0/DIO0" ("APD 1 DO"), "Timeout"=-1) -> ()  [unwired: 2 out]
      }
      frame #1 {
        n217 = xnode "FPGA I/O Node"() -> ("Connector0/DIO9"=w440:bool, "Connector0/DIO6"=w439:bool)  [unwired: 2 in, 2 out]
        n218 = case shown="True" w440 {
          tunnel: w442 -> [_ w445]
          tunnel: [u32 0 w444] -> w441
          tunnel: w439 -> [_ w447]
          tunnel: w438 -> [_ w446]
          frame False {
          }
          frame True {
            n219 = case shown="True" w447 {
              tunnel: w446 -> [w450 w455]
              tunnel: w445 -> [w449 w456]
              tunnel: [w448 w454] -> w444
              frame False {
                n220 = case shown="True" w450 {
                  tunnel: w449 -> [w452 _]
                  tunnel: [w451 u32 1] -> w448
                  frame False {
                    n221 = Increment(x=w452) -> (x+1=w451:u32)
                  }
                  frame True {
                  }
                }
                "APD 1 Counts 0" <- w448
              }
              frame True {
                n222 = case shown="True" w455 {
                  tunnel: w456 -> [_ w459]
                  tunnel: [u32 1 w458] -> w454
                  frame False {
                  }
                  frame True {
                    n223 = Increment(x=w459) -> (x+1=w458:u32)
                  }
                }
                "APD 1 Counts 1" <- w454
              }
            }
          }
        }
      }
    }
  }
  n224 = while "RF synth board interlacing timing loop" {
    tunnel: w2 -> [_]
    stop <- FALSE stop-if-true
    # "This loop is stalled until the RF FIFO get a value. With this method we gain additional delay time (because  we allow the rest of the main RF loop to procede while this loop waits to send the switch signals - a form of parallelism). This helps to simplify the main RF code. \n\nThe code also allow optimal interlacing while also controlling trap RF phase. \n\nNote: a lot of work has gone into optimizing these methods and it is unclear how they can be made any faster or better than this (many failed tries). Right now there is essentially ~4 ticks (~90 ns ns) of imperfection in the switching from trap 1 to trap 2. ~2 ticks of no RF (phase reset) then ~2 ticks of trap 2 with the wrong amplitude (T1 amplitude). The total ticks is 200, so not a big error.\n\nPhase can be precisely set for each trap. Phase reset and switching, has similar delays as fsk frequency switching. And phase reset and phase offset changes are also not simultaneous. So we can't perfectly line everything up.\n\nIf you start from amp zero though (as for trap 1), the on switch is perfect. Likewise the off is perfect for trap 2. \n\nThe green laser switching is also perfect because of its reduced duty cycle and delays in fsk switching between 80 and 0 MHz."
    n225 = xnode ("FIFO Read")("Timeout"=-1) -> ("Element"=w506:u16, "FIFO Out"=w502:refnum<k21>)  [unwired: 1 in, 1 out]
    n226 = Equal To 0?(x=w506) -> (x = 0?=w503:bool)
    n227 = Not(x=w503) -> (.not. x?=w460:bool)
    n228 = flat-sequence "BD 1 and 2 RF phase and amplitude switching" {
      tunnel: w460 -> [_]
      tunnel: w495 -> [w610]
      tunnel: w494 -> [w609]
      tunnel: w493 -> [w608]
      tunnel: w492 -> [w607]
      tunnel: w491 -> [w606]
      tunnel: w490 -> [w605]
      tunnel: w489 -> [w604]
      tunnel: w488 -> [w603]
      tunnel: w486 -> [w602]
      tunnel: w485 -> [w601]
      tunnel: w484 -> [w600]
      tunnel: w482 -> [w598]
      tunnel: w481 -> [w597]
      tunnel: w480 -> [w596]
      tunnel: w483 -> [w599]
      tunnel: w487 -> [w595]
      tunnel: w479 -> [w634]
      tunnel: w478 -> [w633]
      tunnel: w477 -> [w632]
      tunnel: w476 -> [w631]
      tunnel: w475 -> [w630]
      tunnel: w474 -> [w629]
      tunnel: w473 -> [w628]
      tunnel: w472 -> [w627]
      tunnel: w471 -> [w626]
      tunnel: w469 -> [w625]
      tunnel: w468 -> [w624]
      tunnel: w467 -> [w623]
      tunnel: w466 -> [w622]
      tunnel: w465 -> [w621]
      tunnel: w464 -> [w620]
      tunnel: w470 -> [w619]
      frame #0 {
        # "Delay to align amp/frequency switching depending on the method used.\n\nCan also give enough time to do the parallel amplitude calculations"
        n229 = call "Wait2"("Count(Ticks)"="Amp switch delay") -> ()  [unwired: 1 out]
      }
      frame #1 {
        w590 = TRUE ("Connector1/DIO30")
        # "make phase offset and phase reset active with buffer transfer"
        n230 = xnode "FPGA I/O Node"("Connector1/DIO29"=w590, "Connector1/DIO30"=w590) -> ()  [unwired: 2 in, 2 out]
      }
      frame #2 {
        w591 = FALSE ("Connector1/DIO15")
        # "write phase restart to buffer and reset udclk"
        n231 = xnode "FPGA I/O Node"("Connector1/DIO29"=w591, "Connector1/DIO30"=w591, "Connector1/DIO15"=FALSE ("Connector1/DIO14")) -> ()  [unwired: 3 in, 3 out]
      }
      frame #3 {
        w593 = TRUE ("Connector1/DIO15")
        # "make phase restart active"
        # "reset WR"
        n232 = xnode "FPGA I/O Node"("Connector1/DIO15"=w593, "Connector1/DIO29"=w593, "Connector1/DIO30"=w593) -> ()  [unwired: 3 in, 3 out]
      }
      frame #4 {
        w594 = FALSE ("Connector1/DIO30")
        # "Address"
        # "set amp byte 1, and reset udclk"
        n233 = xnode "FPGA I/O Node"("Connector1/DIO0"=w610, "Connector1/DIO1"=w609, "Connector1/DIO2"=w608, "Connector1/DIO3"=w607, "Connector1/DIO4"=w606, "Connector1/DIO5"=w605, "Connector1/DIO6"=w604, "Connector1/DIO7"=w603, "Connector1/DIO8"=TRUE, "Connector1/DIO9"=FALSE, "Connector1/DIO10"=FALSE, "Connector1/DIO11"=FALSE, "Connector1/DIO12"=FALSE, "Connector1/DIO13"=TRUE, "Connector1/DIO20"=w595, "Connector1/DIO21"=w602, "Connector1/DIO22"=w601, "Connector1/DIO23"=w600, "Connector1/DIO24"=w599, "Connector1/DIO25"=w598, "Connector1/DIO26"=w597, "Connector1/DIO27"=w596, "Connector1/DIO30"=w594, "Connector1/DIO29"=w594) -> ()  [unwired: 24 in, 24 out]
      }
      frame #5 {
        # "write amp byte 1 to buffer"
        n234 = xnode "FPGA I/O Node"("Connector1/DIO15"=FALSE ("Connector1/DIO14")) -> ()  [unwired: 1 in, 1 out]
      }
      frame #6 {
        # "reset WR"
        n235 = xnode "FPGA I/O Node"("Connector1/DIO15"=TRUE) -> ()  [unwired: 1 in, 1 out]
      }
      frame #7 {
        # "Address"
        # "set amp byte 2"
        n236 = xnode "FPGA I/O Node"("Connector1/DIO0"=w634, "Connector1/DIO1"=w633, "Connector1/DIO2"=w632, "Connector1/DIO3"=w631, "Connector1/DIO4"=w630, "Connector1/DIO5"=w629, "Connector1/DIO6"=w628, "Connector1/DIO7"=w627, "Connector1/DIO8"=TRUE, "Connector1/DIO9"=FALSE, "Connector1/DIO10"=FALSE, "Connector1/DIO11"=FALSE, "Connector1/DIO12"=TRUE, "Connector1/DIO13"=FALSE, "Connector1/DIO20"=w626, "Connector1/DIO21"=w619, "Connector1/DIO22"=w625, "Connector1/DIO23"=w624, "Connector1/DIO24"=w623, "Connector1/DIO25"=w622, "Connector1/DIO26"=w621, "Connector1/DIO27"=w620) -> ()  [unwired: 22 in, 22 out]
      }
      frame #8 {
        # "write amp byte 2"
        n237 = xnode "FPGA I/O Node"("Connector1/DIO15"=FALSE ("Connector1/DIO14")) -> ()  [unwired: 1 in, 1 out]
      }
      frame #9 {
        w642 = TRUE ("Connector1/DIO15")
        # "transfer amp bytes 1 and 2 and reset WR"
        n238 = xnode "FPGA I/O Node"("Connector1/DIO29"=w642, "Connector1/DIO30"=w642, "Connector1/DIO15"=TRUE ("Connector1/DIO14")) -> ()  [unwired: 3 in, 3 out]
      }
      frame #10 {
        w644 = FALSE ("Connector1/DIO14")
        # "reset udclk"
        n239 = xnode "FPGA I/O Node"("Connector1/DIO29"=w644, "Connector1/DIO30"=w644) -> ()  [unwired: 2 in, 2 out]
      }
    }
    n240 = flat-sequence "FSK BD 1 (trap X)" {
      tunnel: w460 -> [w508]
      tunnel: [w508] -> w463
      tunnel: w463 -> [w509]
      frame #0 {
        n241 = call "Wait"("Count(Ticks)"="BD 1 Delay (ticks)") -> ()  [unwired: 1 out]
      }
      frame #1 {
        # "switch frequency"
        n242 = xnode "FPGA I/O Node"("Connector1/DIO36"=w509) -> ()  [unwired: 1 in, 1 out]
      }
    }
    n243 = flat-sequence "FSK BD 2 (trap Y or green laser AOM)" {
      tunnel: w460 -> [w646]
      tunnel: [w646] -> w505
      tunnel: w505 -> [w647]
      frame #0 {
        n244 = call "Wait3"("Count(Ticks)"="BD 2 Delay (Ticks)") -> ()  [unwired: 1 out]
      }
      frame #1 {
        # "switch frequency"
        n245 = xnode "FPGA I/O Node"("Connector1/DIO37"=w647) -> ()  [unwired: 1 in, 1 out]
      }
    }
    n246 = xnode ("FIFO Read")("Timeout"=-1, "FIFO In"=w502) -> ("Element"=w497:u16, "FIFO Out"=w501:refnum<k21>)  [unwired: 1 out]
    n247 = xnode ("FIFO Read")("Timeout"=-1, "FIFO In"=w501) -> ("Element"=w496:u16)  [unwired: 2 out]
    n248 = node-c288() -> (w499:T7)  [unwired: 1 in]
    n249 = timed-loop "Convert amplitude words to bits" {
      timing: w499 -> [_]
      timing-out: [_] -> w498
      tunnel: w497 -> [w566]
      tunnel: w496 -> [w565]
      tunnel: [w542] -> w495
      tunnel: [w541] -> w494
      tunnel: [w540] -> w493
      tunnel: [w539] -> w492
      tunnel: [w538] -> w491
      tunnel: [w537] -> w490
      tunnel: [w536] -> w489
      tunnel: [w535] -> w488
      tunnel: [w534] -> w487
      tunnel: [w533] -> w486
      tunnel: [w532] -> w485
      tunnel: [w531] -> w484
      tunnel: [w530] -> w483
      tunnel: [w529] -> w482
      tunnel: [w528] -> w481
      tunnel: [w527] -> w480
      tunnel: [w526] -> w479
      tunnel: [w525] -> w478
      tunnel: [w524] -> w477
      tunnel: [w523] -> w476
      tunnel: [w522] -> w475
      tunnel: [w521] -> w474
      tunnel: [w520] -> w473
      tunnel: [w519] -> w472
      tunnel: [w518] -> w471
      tunnel: [w517] -> w470
      tunnel: [w516] -> w469
      tunnel: [w515] -> w468
      tunnel: [w514] -> w467
      tunnel: [w513] -> w466
      tunnel: [w512] -> w465
      tunnel: [w511] -> w464
      stop <- TRUE stop-if-true
      # "Board 1 Data"
      # "Board 2 Data"
      # "Board 1 Data"
      # "Board 2 Data"
      n250 = Split Number(x=w566) -> (hi(x)=w564:u8, lo(x)=w544:u8)
      n251 = Split Number(x=w565) -> (hi(x)=w563:u8, lo(x)=w543:u8)
      n252 = Number To Boolean Array(number=w564) -> (Boolean array=w584:bool[])
      n253 = Number To Boolean Array(number=w563) -> (Boolean array=w575:bool[])
      n254 = Index Array(array=w584, index=7) -> (element=w542:bool)
      n255 = Index Array(array=w584, index=6) -> (element=w541:bool)
      n256 = Index Array(array=w584, index=5) -> (element=w540:bool)
      n257 = Index Array(array=w584, index=4) -> (element=w539:bool)
      n258 = Index Array(array=w584, index=3) -> (element=w538:bool)
      n259 = Index Array(array=w584, index=2) -> (element=w537:bool)
      n260 = Index Array(array=w584, index=1) -> (element=w536:bool)
      n261 = Index Array(array=w584, index=0) -> (element=w535:bool)
      n262 = Index Array(array=w575, index=7) -> (element=w534:bool)
      n263 = Index Array(array=w575, index=6) -> (element=w533:bool)
      n264 = Index Array(array=w575, index=5) -> (element=w532:bool)
      n265 = Index Array(array=w575, index=4) -> (element=w531:bool)
      n266 = Index Array(array=w575, index=3) -> (element=w530:bool)
      n267 = Index Array(array=w575, index=2) -> (element=w529:bool)
      n268 = Index Array(array=w575, index=1) -> (element=w528:bool)
      n269 = Index Array(array=w575, index=0) -> (element=w527:bool)
      n270 = Number To Boolean Array(number=w544) -> (Boolean array=w562:bool[])
      n271 = Number To Boolean Array(number=w543) -> (Boolean array=w553:bool[])
      n272 = Index Array(array=w562, index=7) -> (element=w526:bool)
      n273 = Index Array(array=w562, index=6) -> (element=w525:bool)
      n274 = Index Array(array=w562, index=5) -> (element=w524:bool)
      n275 = Index Array(array=w562, index=4) -> (element=w523:bool)
      n276 = Index Array(array=w562, index=3) -> (element=w522:bool)
      n277 = Index Array(array=w562, index=2) -> (element=w521:bool)
      n278 = Index Array(array=w562, index=1) -> (element=w520:bool)
      n279 = Index Array(array=w562, index=0) -> (element=w519:bool)
      n280 = Index Array(array=w553, index=7) -> (element=w518:bool)
      n281 = Index Array(array=w553, index=6) -> (element=w517:bool)
      n282 = Index Array(array=w553, index=5) -> (element=w516:bool)
      n283 = Index Array(array=w553, index=4) -> (element=w515:bool)
      n284 = Index Array(array=w553, index=3) -> (element=w514:bool)
      n285 = Index Array(array=w553, index=2) -> (element=w513:bool)
      n286 = Index Array(array=w553, index=1) -> (element=w512:bool)
      n287 = Index Array(array=w553, index=0) -> (element=w511:bool)
    }
    n288 = node-c288(w498) -> ()
  }
  n289 = while "APD  Gating" {
    shift-right: [w651] -> _
    shift-left: w2 -> [w656]
    shift-right: [w650] -> _
    shift-left: FALSE -> [w648]
    stop <- FALSE stop-if-true
    n290 = flat-sequence {
      tunnel: w656 -> [w659]
      tunnel: [w660] -> w654
      tunnel: [w659] -> w652
      tunnel: [w658] -> w649
      tunnel: w648 -> [w658]
      tunnel: [w663] -> w655
      tunnel: w654 -> [w663]
      tunnel: [w662] -> w653
      tunnel: w652 -> [w662]
      tunnel: w649 -> [w661]
      tunnel: [w681] -> w651
      tunnel: w655 -> [w695]
      tunnel: w653 -> [w692]
      tunnel: [w664] -> w650
      frame #0 {
        n291 = call "Loop Timer4"("Count(Ticks)"=w659) -> ("Tick Count(Ticks)"=w660:u32)
      }
      frame #1 {
        # "Signal maybe then sent through \na transistor before APD"
        n292 = xnode "FPGA I/O Node"("Connector1/DIO33"=w661, "Connector0/DIO7"=w661) -> ()  [unwired: 2 in, 2 out]
      }
      frame #2 {
        n293 = feedback #20(TRUE) -> (w687:bool)
        n294 = feedback-in #21(w695) -> ()
        n295 = feedback #21(w695) -> (w694:u32)
        n296 = Not(x=w687) -> (.not. x?=w684:bool)
        n297 = feedback-in #20(w684) -> ()
        n298 = Subtract(x=w695, y=w694) -> (x-y=w693:u32)
        n299 = Select(t="APD Gate ON Count", s=w684, f="APD Gate OFF Count") -> (s? t:f=w689:u16)
        n300 = Subtract(x=w693, y=w692) -> (x-y=w669:u32)
        n301 = Subtract(x=w689, y=w669) -> (x-y=w680:u32)
        n302 = Number To Boolean Array(number=w669) -> (Boolean array=w670:bool[])
        n303 = Or Array Elements(Boolean array=w670) -> (logical OR=w668:bool)
        n304 = Boolean To (0,1)(Boolean="+ phase (APD 1 Gate)") -> (0, 1=w678:i16)
        n305 = Boolean To (0,1)(Boolean=w668) -> (0, 1=w675:i16)
        n306 = Multiply(x=w678, y="Phase count adjustment (APD 1 Gate)") -> (x*y=w676:i16)
        n307 = To Unsigned Byte Integer(number=w675) -> (unsigned 8bit integer=w672:u8)
        n308 = Add(x=w680, y=w676) -> (x+y=w681:u32)
        n309 = feedback #22(i16 0) -> (w683:i16)
        n310 = Subtract(x=w683, y=w676) -> (x-y=w682:i16)
        "APD 1 Gate Relative Phase" <- w682
        n311 = feedback-in #22(w682) -> ()
        n312 = feedback #23(u8 0) -> (w673:u8)
        n313 = Add(x=w672, y=w673) -> (x+y=w671:u8)
        "APD 1 Gate Late Counter" <- w671
        n314 = feedback-in #23(w671) -> ()
        n315 = case shown="2" "APD Gate Operating Mode" {
          tunnel: [TRUE FALSE w698] -> w665
          tunnel: w687 -> [_ _ w698]
          frame 0, Default {
          }
          frame 1 {
          }
          frame 2 {
          }
        }
        n316 = Not(x=w665) -> (.not. x?=w666:bool)
        n317 = Select(t=w666, s="Invert APD Gate", f=w665) -> (s? t:f=w664:bool)
      }
    }
  }
  n318 = while "Trap RF control, main calculations (raster scanning, intensity and position feedback, phase control etc) with primary timing trigger" {
    shift-right: [w713] -> _
    shift-left: w2 -> [w712]
    shift-right: [w711] -> _
    shift-left: FALSE ("Swap F1 and F2") -> [w710]
    shift-right: [w706] -> _
    shift-left: u16 0 ("BD 1 Amplitude 3") -> [w703]
    shift-right: [w705] -> _
    shift-left: u16 0 ("BD 2 Amplitude 3") -> [w701]
    shift-right: [w700] -> _
    shift-left: u64 0 -> [w699]
    stop <- FALSE stop-if-true
    n319 = flat-sequence {
      tunnel: w710 -> [w719]
      tunnel: w712 -> [w716]
      tunnel: [w719] -> w709
      tunnel: [w715] -> w708
      tunnel: [w716] -> w707
      tunnel: [w718] -> w704
      tunnel: w703 -> [w718]
      tunnel: [w717] -> w702
      tunnel: w701 -> [w717]
      tunnel: [w730] -> w713
      tunnel: [w729] -> w711
      tunnel: w709 -> [w728]
      tunnel: w708 -> [w727]
      tunnel: w707 -> [w726]
      tunnel: [w725] -> w706
      tunnel: [w724] -> w705
      tunnel: w704 -> [w723]
      tunnel: w702 -> [w722]
      tunnel: [w721] -> w700
      tunnel: w699 -> [w720]
      frame #0 {
        n320 = call "Loop Timer2"("Count(Ticks)"=w716) -> ("Tick Count(Ticks)"=w715:u32)
      }
      frame #1 {
        n321 = flat-sequence {
          tunnel: w728 -> [w738]
          tunnel: w723 -> [w732]
          tunnel: w722 -> [w731]
          tunnel: [w798] -> w730
          tunnel: [w810] -> w729
          tunnel: w727 -> [w804]
          tunnel: w726 -> [w801]
          tunnel: [w749] -> w725
          tunnel: [w748] -> w724
          tunnel: [w740] -> w721
          tunnel: w720 -> [w739]
          frame #0 {
            w733 = -1 ("Timeout")
            # "Operation when you need a long delay for either X or Y to synchonize AOD light out phase (> ~100 ticks)\nor want shorter trap ON timing. Puts some of the delay timing in parallel with the later computations."
            # "Trigger the external loop by sending the boolean FSK value through a FIFO.\nTiming is precise."
            n322 = Boolean To (0,1)(Boolean=w738) -> (0, 1=w737:i16)
            n323 = To Unsigned Word Integer(number=w737) -> (unsigned 16bit integer=w736:u16)
            n324 = xnode ("FIFO Method Node")("Element"=w736, "Timeout"=w733) -> ("FIFO Out"=w735:refnum<k21>)  [unwired: 1 in, 1 out]
            n325 = xnode ("FIFO Method Node")("Element"=w732, "Timeout"=w733, "FIFO In"=w735) -> ("FIFO Out"=w734:refnum<k21>)  [unwired: 1 out]
            n326 = xnode ("FIFO Method Node")("Element"=w731, "Timeout"=w733, "FIFO In"=w734) -> ()  [unwired: 2 out]
          }
          frame #1 {
            # "Just counts, wraps around, 8 bit"
            # "Which trap cycle"
            # "Only save the 3rd set's amp in the loop"
            # "If this is NOT set 3 AND NOT (RF synth controls green AND green FB running)\nthen use this sets amp value (otherwise keep the green feedback value)"
            # "Just flips back and forth."
            # "If interlacing is off, this is which cycle to use."
            # "Keep track of trap cycles (trap 1, 2, 3...)"
            # "This is the prior cycle's on time"
            # "increment timing\nindex, reset to 0 if \nend of matrix"
            # "Reset to begginning (1) when number of cycles reached."
            # "timing index"
            # "build byte stacks for writing data\n(must correspond to addresses array constant)"
            # "Timing housekeeping"
            # "Adjust phase if late\n(maintains constant phase relationship between cycles)"
            n327 = feedback #24(u8 0 ("t")) -> (w807:u8)
            n328 = Increment(x=w807) -> (x+1=w846:u8)
            n329 = Increment(x="Number Interlace Cycles") -> (x+1=w841:u8)
            n330 = Equal?(x=w846, y=w841) -> (x = y?=w848:bool)
            n331 = Select(t=u8 1, s=w848, f=w846) -> (s? t:f=w806:u8)
            n332 = feedback-in #24(w806) -> ()
            n333 = Increment(x=w806) -> (x+1=w843:u8)
            n334 = Equal?(x=w843, y=w841) -> (x = y?=w844:bool)
            n335 = Select "This cycle"(t=u8 1, s=w844, f=w843) -> (s? t:f=w840:u8)
            n336 = Select(t=w840, s="Interlace ON/OFF", f="Interlace Off Parameters") -> (s? t:f=w759:u8)
            n337 = feedback-in #25(w804) -> ()
            n338 = feedback #25(w804) -> (w803:u32)
            n339 = Select(t=w806, s="Interlace ON/OFF", f="Interlace Off Parameters") -> (s? t:f=w839:u8)
            n340 = Subtract(x=w804, y=w803) -> (x-y=w802:u32)
            n341 = Subtract "The error"(x=w802, y=w801) -> (x-y=w785:u32)
            n342 = case shown="1, Default" w839 {
              tunnel: ["DIO count 1 (ticks)" "DIO count 2 (ticks)" "DIO count 3 (ticks)"] -> w800
              frame 1, Default {
              }
              frame 2 {
              }
              frame 3 {
              }
            }
            n343 = Number To Boolean Array(number=w785) -> (Boolean array=w786:bool[])
            n344 = Or Array Elements(Boolean array=w786) -> (logical OR=w784:bool)
            n345 = Boolean To (0,1)(Boolean=w784) -> (0, 1=w791:i16)
            n346 = To Unsigned Byte Integer(number=w791) -> (unsigned 8bit integer=w788:u8)
            n347 = feedback #26(u8 0) -> (w789:u8)
            n348 = Add(x=w788, y=w789) -> (x+y=w787:u8)
            "DIO Late Counter" <- w787
            n349 = feedback-in #26(w787) -> ()
            n350 = Subtract(x=w800, y=w785) -> (x-y=w799:u32)
            n351 = disable-structure shown="Disabled" {
              disable-tunnel: [w852 _] -> w783
              disable-tunnel: w759 -> [w849 _]
              frame Disabled {
                n352 = feedback #27(i64 0 ("y")) -> (w851:i64)
                n353 = case "Synchronize trap oscillations - always begin/end with trap 1" shown="1, Default" w849 {
                  tunnel: [w853 w854 w855] -> w852
                  tunnel: w851 -> [w853 w854 _]
                  frame 2 {
                  }
                  frame 3 {
                  }
                  frame 1, Default {
                    n354 = Or(x="Osc traps", y="Initiate trap osc") -> (x .or. y?=w857:bool)
                    n355 = case "Trap sine oscillation (or whatever pattern is stored in memory)" shown="True" w857 {
                      tunnel: [i64 0 ("y") w861] -> w855
                      tunnel: "Initiate trap osc" -> [_ w864]
                      frame False {
                      }
                      frame True {
                        w868 = u16 0
                        w866 = -1
                        n356 = local write "Initiate trap osc"(FALSE ("Initiate trap osc")) -> ()
                        n357 = feedback #28(w868) -> (w870:u16)
                        n358 = Select(t=w868, s=w864, f=w870) -> (s? t:f=w869:u16)
                        n359 = Greater Or Equal?(x=w869, y="Trap osc period (pts)") -> (x >= y?=w875:bool)
                        n360 = Or(x=w864, y=w875) -> (x .or. y?=w876:bool)
                        n361 = Select(t=u16 0, s=w876, f=w869) -> (s? t:f=w860:u16)
                        n362 = feedback #29(w866) -> (w867:i32)
                        n363 = Select(t=w866, s=w864, f=w867) -> (s? t:f=w865:i32)
                        n364 = Increment(x=w865) -> (x+1=w872:i32)
                        n365 = Equal?(x=w860, y=u16 0) -> (x = y?=w873:bool)
                        n366 = Increment(x=w860) -> (x+1=w880:u16)
                        n367 = feedback-in #28(w880) -> ()
                        n368 = Select(t=w872, s=w873, f=w865) -> (s? t:f=w871:i32)
                        n369 = feedback-in #29(w871) -> ()
                        n370 = case shown="False" "Osc trap cont." {
                          tunnel: w871 -> [w884 _]
                          frame False {
                            n371 = Greater Or Equal?(x=w884, y="N trap osc periods") -> (x >= y?=w882:bool)
                            n372 = Not(x=w882) -> (.not. x?=w881:bool)
                            n373 = local write "Osc traps"(w881) -> ()
                          }
                          frame True {
                          }
                        }
                        n374 = xnode ("Memory Read")("Address"=w860, "Memory In"=refnum<k21> "Trap osc memory") -> ("Data"=w861:i64)  [unwired: 1 out]
                      }
                    }
                  }
                }
                n375 = feedback-in #27(w852) -> ()
              }
              frame Enabled {
              }
            }
            n376 = local read "green FB running"() -> (w772:bool)
            n377 = And(x=w772, y="RF synth bd controls green") -> (x .and. y?=w771:bool)
            n378 = case shown="1, Default" w759 {
              tunnel: [w1011 w1247 "BD 1 Frequency 3"] -> w836
              tunnel: [w1052 w1246 w1268] -> w775
              tunnel: ["BD 2 Amplitude 1" "BD 2 Amplitude 2" w1267] -> w767
              tunnel: [w1008 w1243 "BD 1 Amplitude 3"] -> w749
              tunnel: "FB Gains" -> [w1029 w1253 _]
              tunnel: "FB output range" -> [w1030 w1252 _]
              tunnel: w783 -> [w1027 w1250 _]
              tunnel: "BD 2 Frequency 1" -> [w1024 _ _]
              tunnel: "BD 2 Frequency 2" -> [_ w1246 _]
              tunnel: "BD 2 Frequency 3" -> [_ _ w1268]
              tunnel: w771 -> [_ _ w1266]
              tunnel: [w1011 w1244 w1265] -> w740
              tunnel: w739 -> [w1010 w1244 w1265]
              frame 1, Default {
                w1043 = fxp<+/-,24,9> 0.0 ("AI1 X Set 2")
                w1037 = u16 0
                w1050 = u64 0 ("f")
                # "% Intensity feedback.... is not really \"feedback\" - the PID _change_ is set to the amplitude _position_\n....this ends up working ok? but thats why ur set point (V) isn't your actual laser power (V)\n\nthis does presumably use less FPGA resources,  and works just about as well as a proper implementation\n  (the response is still quite linear), just is really weird to see --Alex 081418"
                # "Changed by Ronen - correction \nby PID is now implemented not on \nthe Base BD1 frequency but on the last\nfrequency sent."
                # "Added by Ronen -\nUpper and Lower \nLimits for the FB \ngenerated frequency\nto avoid losing bead \nwhen tether breaks"
                # "Explanation of raster scanning:\n1. Cycles: increment counter by 1 every time interlace cycle returns to trap 1. As long as \n  Cycle per Step is larger than counter, keep incrementing counter and do not change step counter.\n  Once counter is equal to Cycles per step, zero counter and increment step counter.\n2. Steps: Increments up every time cycles counter equals cycles per step. Performs the following:\n- To determine DIRECTION of frequency change:  If ScanstepX2 is EQUAL to step counter (full for-back scan finished)\n   frequency increment is set to zero, AND step counter is set to zero. \n   Otherwise: if no change to step counter (because cycleperstep>cycle counter), then no change to frequency\n   increment. \n   If step counter has changed (cycleperstep=cycle counter), then need to figure out direction of frequency change:\n   if step counter is EQUAL to Scansteps: No change to frequency increment\n   Otherwise: If scan steps > step counter - 1 (forward scan NOT completed): increment frequency by 1\n                       If scan steps equal or smaller than step counter -1 (forward scan completed): increment frequency by -1\n\n3. Scans: Increment scan counter every time step counter equals 2Xscan steps (full for-back scan completed)\n    if number of scans > scan counter: Send TRUE to scanning, continue scan\n    if number of scans = scan counter: Send FALSE to Scanning, Scan finished.\n\n  The wire with the asterik can be used as the index for getting the mirror positions in the offset scan."
                # "This signal integration happens no matter what\nso that correct setpoints can be chosen before \nturning on the FB."
                # "Trap 1"
                n379 = local read "AI1 X Set 2"() -> (w1022:fxp<+/-,16,1>)
                n380 = local read "AI1 X Set 1"() -> (w1040:fxp<+/-,16,1>)
                n381 = local read "Scanning"() -> (w1053:bool)
                n382 = Multiply(x=w1022, y="B factor") -> (x*y=w1020:fxp<+/-,48,17>)
                n383 = Or(x=w1053, y="Start scan") -> (x .or. y?=w1005:bool)
                n384 = case shown="True" "Diff FB Measurement?" {
                  tunnel: w1020 -> [w1143 w1152]
                  tunnel: w1040 -> [w1142 w1153]
                  tunnel: [w1140 w1144] -> w1041
                  frame False {
                    n385 = Select(t=w1142, s="Trap Pos FB Monitor T1 or T2", f=w1143) -> (s? t:f=w1140:fxp<+/-,48,17>)
                  }
                  frame True {
                    n386 = Subtract(x=w1153, y=w1152) -> (x-y=w1145:fxp<+/-,48,17>)
                    n387 = Not(x="Negate Diff?") -> (.not. x?=w1151:bool)
                    n388 = Boolean To (0,1)(Boolean="Negate Diff?") -> (0, 1=w1149:i16)
                    n389 = Boolean To (0,1)(Boolean=w1151) -> (0, 1=w1150:i16)
                    n390 = Negate(x=w1149) -> (-x=w1148:i16)
                    n391 = Add(x=w1148, y=w1150) -> (x+y=w1146:i16)
                    n392 = Multiply(x=w1146, y=w1145) -> (x*y=w1144:fxp<+/-,63,32>)
                  }
                }
                n393 = feedback #30(w1037) -> (w1036:u16)
                n394 = Increment(x=w1036) -> (x+1=w1038:u16)
                n395 = Greater Or Equal?(x=w1038, y="Trap Pos FB Int Count") -> (x >= y?=w1009:bool)
                n396 = Select(t=w1037, s=w1009, f=w1038) -> (s? t:f=w1039:u16)
                n397 = feedback-in #30(w1039) -> ()
                n398 = feedback #31(w1043) -> (w1042:fxp<+/-,24,9>)
                n399 = Add(x=w1041, y=w1042) -> (x+y=w1035:fxp<+/-,24,9>)
                n400 = Select(t=w1043, s=w1009, f=w1035) -> (s? t:f=w1046:fxp<+/-,24,9>)
                n401 = feedback-in #31(w1046) -> ()
                n402 = case "Trap 1 X intensity feedback" shown="True" "FB On/Off Set 1" {
                  tunnel: "BD 1 Amplitude 1" -> [w1235 _]
                  tunnel: [w1235 w1239] -> w1008
                  tunnel: w1030 -> [_ w1236]
                  tunnel: w1029 -> [_ w1237]
                  frame False {
                  }
                  frame True {
                    n403 = local read "AI2 Y Sum Set 1"() -> (w1240:i16)
                    n404 = call "Slower PID.vi"("process variable"=w1240, "reset?"="FB Reset Set 1", "setpoint"="FB Setpoint Set 1", "PID gains (x 2^8)"=w1237, "output range"=w1236) -> ("output"=w1241:i16)  [unwired: 10 out]
                    n405 = To Unsigned Word Integer(number=w1241) -> (unsigned 16bit integer=w1239:u16)
                  }
                }
                "BD1 amplitude 1 out" <- w1008
                n406 = Divide(x=w1035, y="Trap Pos FB Int Count") -> (x/y=w1006:fxp<+/-,16,1>)
                n407 = case "For raster scanning" shown="True" w1005 {
                  tunnel: [u64 0 w1083] -> w1007
                  tunnel: [FALSE w1071] -> w1000
                  tunnel: [i16 0 w1070] -> w1001
                  tunnel: w1006 -> [_ w1069]
                  tunnel: "Start scan" -> [_ w1063]
                  frame False {
                    n408 = local write "Scanning"(FALSE ("scanning")) -> ()
                  }
                  frame True {
                    w1077 = u64 0
                    # "Changed by RG, to introduce force\ndependent stopping of the raster scan \nand manual stopping"
                    # "count number of cycles"
                    n409 = feedback #32(w1077) -> (w1080:u64)
                    n410 = Select(t=w1077, s=w1063, f=w1080) -> (s? t:f=w1082:u64)
                    n411 = Increment(x=w1082) -> (x+1=w1075:u64)
                    n412 = Equal?(x=i16 1, y=w1075) -> (x = y?=w1073:bool)
                    n413 = And(x="Abort scan", y=w1073) -> (x .and. y?=w1071:bool)
                    n414 = Greater?(x="Cycles per step", y=w1075) -> (0:w1078:bool)
                    n415 = Select(t=w1075, s=w1078, f=w1077) -> (s? t:f=w1079:u64)
                    n416 = feedback-in #32(w1079) -> ()
                    n417 = Greater?(x=w1069, y="Raster setpoint") -> (0:w1066:bool)
                    n418 = And(x=w1066, y="Raster to target force") -> (x .and. y?=w1064:bool)
                    n419 = case shown="False" w1071 {
                      tunnel: [w1090 i16 0] -> w1083
                      tunnel: w1063 -> [w1115 _]
                      tunnel: w1078 -> [w1108 _]
                      tunnel: w1077 -> [w1098 _]
                      tunnel: [w1092 FALSE] -> w1072
                      tunnel: [w1088 w1126] -> w1070
                      tunnel: [w1091 w1127] -> w1067
                      frame False {
                        w1099 = i64 0
                        # "scan incr."
                        # "freq. incr. mult."
                        # "count steps"
                        n420 = feedback #33(w1098) -> (w1123:u64)
                        n421 = Select(t=w1098, s=w1115, f=w1123) -> (s? t:f=w1091:u64)
                        n422 = Increment(x=w1091) -> (x+1=w1122:u64)
                        n423 = Add(x="Scan steps", y="Scan steps") -> (x+y=w1121:u64)
                        n424 = Select(t=w1091, s=w1108, f=w1122) -> (s? t:f=w1103:u64)
                        n425 = Greater?(x=w1121, y=w1103) -> (0:w1102:bool)
                        n426 = Select(t=w1103, s=w1102, f=w1098) -> (s? t:f=w1119:u64)
                        n427 = feedback-in #33(w1119) -> ()
                        n428 = Equal?(x="Scan steps", y=w1103) -> (x = y?=w1107:bool)
                        n429 = Greater?(x="Scan steps", y=w1091) -> (0:w1118:bool)
                        n430 = feedback #34(w1099) -> (w1120:i64)
                        n431 = Select(t=w1099, s=w1115, f=w1120) -> (s? t:f=w1105:i64)
                        n432 = Increment(x=w1105) -> (x+1=w1117:i64)
                        n433 = Decrement(x=w1105) -> (x-1=w1116:i64)
                        n434 = Select(t=w1117, s=w1118, f=w1116) -> (s? t:f=w1106:i64)
                        n435 = Select(t=w1105, s=w1107, f=w1106) -> (s? t:f=w1104:i64)
                        n436 = Select(t=w1105, s=w1108, f=w1104) -> (s? t:f=w1100:i64)
                        n437 = Select(t=w1100, s=w1102, f=w1099) -> (s? t:f=w1101:i64)
                        n438 = feedback-in #34(w1101) -> ()
                        n439 = feedback #35(w1098) -> (w1114:u64)
                        n440 = Select(t=w1098, s=w1115, f=w1114) -> (s? t:f=w1110:u64)
                        n441 = Increment(x=w1110) -> (x+1=w1111:u64)
                        n442 = Select(t=w1110, s=w1102, f=w1111) -> (s? t:f=w1109:u64)
                        n443 = Greater?(x="Number of scans", y=w1109) -> (0:w1095:bool)
                        n444 = Multiply(x="Scan freq.  increment", y=w1105) -> (x*y=w1090:i64)
                        n445 = Select(t=TRUE, s="Cont. Scan", f=w1095) -> (s? t:f=w1092:bool)
                        n446 = Select(t=w1109, s=w1092, f=w1098) -> (s? t:f=w1112:u64)
                        n447 = feedback-in #35(w1112) -> ()
                        n448 = local read "BD 1 Frequency 1"() -> (w1089:u64)
                        n449 = Increment(x=w1109) -> (x+1=→"Scan I":u64)
                        n450 = Add(x=w1090, y=w1089) -> (x+y=w1088:u64)
                        "Actual Scan freq" <- w1088
                      }
                      frame True {
                        n451 = local read "Actual Scan freq"() -> (w1126:u64)
                        n452 = local read "Scan steps"() -> (w1127:u64)
                      }
                    }
                    "Scanning" <- w1072
                    n453 = case shown="True" w1064 {
                      tunnel: w1067 -> [_ w1087]
                      frame False {
                      }
                      frame True {
                        n454 = Add(x=w1087, y=i16 2) -> (x+y=w1085:u64)
                        n455 = local write "Raster to target force"(FALSE) -> ()
                        n456 = local write "Scan steps"(w1085) -> ()
                      }
                    }
                  }
                }
                n457 = feedback #36(fxp<+/-,24,9> 0.0 ("AI1 X Set 2")) -> (w1047:fxp<+/-,24,9>)
                n458 = Select(t=w1035, s=w1009, f=w1047) -> (s? t:f=w1048:fxp<+/-,24,9>)
                "Trap Pos FB Int Signal" <- w1048
                n459 = feedback-in #36(w1048) -> ()
                n460 = feedback #37(fxp<+/-,16,1> 0.0 ("Trap Pos FB Int-Norm Signal")) -> (w1032:fxp<+/-,16,1>)
                n461 = Select(t=w1006, s=w1009, f=w1032) -> (s? t:f=w1031:fxp<+/-,16,1>)
                "Trap Pos FB Int-Norm Signal" <- w1031
                n462 = feedback-in #37(w1031) -> ()
                n463 = case "For position feedback" shown="True" "Force feedback" {
                  tunnel: [i64 0 w1159] -> w1016
                  tunnel: w1006 -> [_ w1156]
                  tunnel: w1009 -> [_ w1155]
                  frame False {
                  }
                  frame True {
                    n464 = feedback #38(i64 0) -> (w1158:i64)
                    n465 = case shown="True" w1155 {
                      tunnel: [w1160 w1164] -> w1159
                      tunnel: w1158 -> [w1160 _]
                      tunnel: w1156 -> [_ w1163]
                      frame False {
                      }
                      frame True {
                        n466 = xnode ("PID")("process variable"=w1163, "reset?"="Trap Pos. FB Reset", "setpoint"="Trap Pos. FB SP", "PID gains"="Trap Pos. FB Gains", "output range"="Trap pos. FB Range") -> ("output"=w1173:fxp<+/-,16,1>)
                        n467 = Negate(x=w1173) -> (-x=w1172:fxp<+/-,17,2>)
                        n468 = Select(t=w1172, s="Trap Pos FB Negate Action", f=w1173) -> (s? t:f=w1169:fxp<+/-,17,2>)
                        n469 = Scale By Power Of 2(n=u32 15, x=u32 1) -> (x*2^n=w1166:u32)
                        n470 = Multiply(x=w1169, y=w1166) -> (x*y=w1165:fxp<+/-,17,17>)
                        n471 = To Quad Integer(1:w1165) -> (0:w1177:i64)
                        "Trap Pos FB Action" <- w1177
                        n472 = Multiply(x=w1177, y="Trap Pos. FB Mult Factor") -> (x*y=w1175:i64)
                        n473 = Add(x=w1175, y="Trap Pos. FB Offset Factor") -> (x+y=w1164:i64)
                        n474 = disable-structure shown="Disabled" {
                          disable-tunnel: w1164 -> [w1184 _]
                          frame Disabled {
                            w1188 = u32 0
                            n475 = feedback #39() -> (w1185:i64)  [unwired: 1 in]
                            n476 = Add(x=w1184, y=w1185) -> (x+y=w1182:i64)
                            n477 = feedback #40(w1188) -> (w1190:u32)
                            n478 = Increment(x=w1190) -> (x+1=w1179:u32)
                            n479 = Greater Or Equal?(x=w1179, y="FB Trig Integrate") -> (x >= y?=w1180:bool)
                            n480 = Select(t=i64 0, s=w1180, f=w1182) -> (s? t:f=w1186:i64)
                            n481 = feedback-in #39(w1186) -> ()
                            n482 = Select(t=w1188, s=w1180, f=w1179) -> (s? t:f=w1189:u32)
                            n483 = feedback-in #40(w1189) -> ()
                            n484 = And(x=w1180, y="FPGA Trap Trig") -> (x .and. y?=w1187:bool)
                            n485 = case "Trap FB trigger excitation laser ON" shown="True" w1187 {
                              tunnel: w1182 -> [_ w1194]
                              tunnel: w1179 -> [_ w1192]
                              frame False {
                              }
                              frame True {
                                n486 = Not(x="TTrig Negate Pos") -> (.not. x?=w1201:bool)
                                n487 = Boolean To (0,1)(Boolean="TTrig Negate Pos") -> (0, 1=w1199:i16)
                                n488 = Boolean To (0,1)(Boolean=w1201) -> (0, 1=w1200:i16)
                                n489 = Negate(x=w1199) -> (-x=w1198:i16)
                                n490 = Add(x=w1198, y=w1200) -> (x+y=w1197:i16)
                                n491 = Multiply(x=w1197, y=w1194) -> (x*y=w1196:i64)
                                "TTrig Sig" <- w1196
                                n492 = Multiply(x="FPGA TTrig Thresh", y=w1192) -> (x*y=w1193:i64)
                                "TTrig Fin Thresh" <- w1193
                                n493 = Greater Or Equal?(x=w1196, y=w1193) -> (x >= y?=w1195:bool)
                                n494 = case shown="True" w1195 {
                                frame False {
                                }
                                frame True {
                                w1204 = TRUE ("Green FB On/Off")
                                w1206 = u8 2 ("Operating Mode")
                                n495 = local write "Operating Mode"(w1206) -> ()
                                n496 = local write item#-1(w1206) -> ()
                                n497 = local write item#-1(w1204) -> ()
                                n498 = local write "FPGA Trap Trig"(FALSE ("FPGA Trap Trig")) -> ()
                                "TTrig?" <- w1204
                                }
                                }
                              }
                            }
                          }
                          frame Enabled {
                          }
                        }
                      }
                    }
                    n499 = feedback-in #38(w1159) -> ()
                  }
                }
                n500 = And(x="Force feedback", y="Dynamic Force FB (Ronen)") -> (x .and. y?=w1017:bool)
                n501 = case shown="False" w1017 {
                  tunnel: w1016 -> [w1131 w1135]
                  tunnel: [w1130 w1134] -> w1002
                  tunnel: w1010 -> [_ w1133]
                  tunnel: w1009 -> [_ w1132]
                  frame False {
                    # "(BD1 Frequency 1)"
                    n502 = Add(x="BD 1 Frequency 1", y=w1131) -> (x+y=w1130:u64)
                  }
                  frame True {
                    n503 = case shown="True" w1132 {
                      tunnel: w1135 -> [_ w1139]
                      tunnel: [w1136 w1138] -> w1134
                      tunnel: w1133 -> [w1136 w1137]
                      frame False {
                      }
                      frame True {
                        n504 = Add(x=w1137, y=w1139) -> (x+y=w1138:u64)
                      }
                    }
                  }
                }
                n505 = case shown="True" w1000 {
                  tunnel: [w1056 w1058] -> w1003
                  tunnel: w1002 -> [w1056 _]
                  tunnel: w1001 -> [_ w1058]
                  frame False {
                  }
                  frame True {
                    n506 = local write "BD 1 Frequency 1"(w1058) -> ()
                    n507 = local write "Abort scan"(FALSE) -> ()
                  }
                }
                n508 = Select(t=w1027, s="Trap 1 osc enable", f=i64 0) -> (s? t:f=w1025:i64)
                n509 = Select(t=w1050, s="Scan BD", f=w1007) -> (s? t:f=w1049:u64)
                n510 = Select(t=w1007, s="Scan BD", f=w1050) -> (s? t:f=w1015:u64)
                n511 = Add(x=w1049, y=w1024) -> (x+y=w1052:u64)
                n512 = Compound Arithmetic op=ADD(w1025, w1003, w1015) -> (w1014:u64)
                n513 = In Range and Coerce(upper limit="FB Max Frequency", x=w1014, lower limit="FB Min frequency") -> (coerced(x)=w1011:u64)  [unwired: 1 out]
                "BD1 Frequency Out 1" <- w1011
              }
              frame 2 {
                # "Trap 2"
                n514 = case "Trap 2 X intensity feedback" shown="True" "FB On/Off Set 2" {
                  tunnel: [w1257 w1260] -> w1243
                  tunnel: "BD 1 Amplitude 2" -> [w1257 _]
                  tunnel: w1253 -> [_ w1259]
                  tunnel: w1252 -> [_ w1258]
                  frame False {
                  }
                  frame True {
                    n515 = local read "AI2 Y Sum Set 2"() -> (w1263:i16)
                    n516 = call "Slower PID.vi"("process variable"=w1263, "reset?"="FB Reset Set 2", "setpoint"="FB Setpoint Set 2", "PID gains (x 2^8)"=w1259, "output range"=w1258) -> ("output"=w1261:i16)  [unwired: 10 out]
                    n517 = To Unsigned Word Integer(number=w1261) -> (unsigned 16bit integer=w1260:u16)
                  }
                }
                "BD1 amplitude 2 out" <- w1243
                n518 = Select(t=w1250, s="Trap 2 osc enable", f=i64 0) -> (s? t:f=w1249:i64)
                n519 = Add(x="BD 1 Frequency 2", y=w1249) -> (x+y=w1247:u64)
                "BD1 Frequency Out 2" <- w1247
              }
              frame 3 {
                # "Fluorescence period"
                n520 = disable-structure shown="Disabled" {
                  disable-tunnel: [w1276 _] -> w1267
                  disable-tunnel: w1266 -> [w1275 _]
                  frame Disabled {
                    # "Remember if FB was previously on/off"
                    n521 = feedback #41(FALSE) -> (w1271:bool)
                    n522 = case shown="True" w1275 {
                      tunnel: [w1278 w1294] -> w1276
                      tunnel: "BD 2 Amplitude 3" -> [w1278 _]
                      tunnel: [FALSE TRUE] -> w1272
                      tunnel: w1271 -> [_ w1280]
                      frame False {
                      }
                      frame True {
                        # "Makes it so first time FB run when turned on, the PID sees the detector intensity from the last time FB was running, rather than something near zero. Especially assuming the setpoint is not changing, this will make the FB more stable when resuming, and not overshoot the turnon intensity."
                        # "FB output range: 0 should be low, full scale is 12 bits.\nBut be careful not to go over, then higher bits just get ignored by RF board, so output will actually jump down and be unstable. Keep it under 4000 to be safe."
                        n523 = local read "Green FB Sum"() -> (w1279:i16)
                        n524 = feedback-in #42(w1279) -> ()
                        n525 = feedback #42(i16 0 ("Green FB Sum")) -> (w1282:i16)
                        n526 = Select(t=w1279, s=w1280, f=w1282) -> (s? t:f=w1281:i16)
                        n527 = Bundle("P3 2"="P3 2", "I3 2"="I3 2", "D3 2"="D3 2") -> (w1293:cluster{"P3 2":i16, "I3 2":i16, "D3 2":i16})  [unwired: 1 in]
                        n528 = Bundle("RF synth green feedback max"="RF synth green feedback max", i16 0) -> (w1285:cluster{"RF synth green feedback max":i16, i16})  [unwired: 1 in]
                        n529 = call "Slower PID.vi"("process variable"=w1281, "reset?"="Green FB Reset 2", "setpoint"="Green FB Setpoint 2", "PID gains (x 2^8)"=w1293, "output range"=w1285) -> ("output"=w1295:i16)  [unwired: 10 out]
                        n530 = To Unsigned Word Integer(number=w1295) -> (unsigned 16bit integer=w1294:u16)
                      }
                    }
                    n531 = feedback-in #41(w1272) -> ()
                  }
                  frame Enabled {
                  }
                }
              }
            }
            n532 = Split Number(x=w836) -> (hi(x)=w835:u32, lo(x)=w834:u32)
            n533 = Boolean To (0,1)(Boolean="+ phase (DIO)") -> (0, 1=w796:i16)
            n534 = Split Number(x=w835) -> (lo(x)=w833:u16)  [unwired: 1 out]
            n535 = Split Number(x=w834) -> (hi(x)=w832:u16, lo(x)=w831:u16)
            n536 = Split Number(x=w833) -> (hi(x)=w825:u8, lo(x)=w824:u8)
            n537 = Split Number(x=w832) -> (hi(x)=w823:u8, lo(x)=w822:u8)
            n538 = Split Number(x=w831) -> (hi(x)=w821:u8, lo(x)=w820:u8)
            n539 = Multiply(x=w796, y="Phase count adjustment (DIO)") -> (x*y=w792:i16)
            n540 = feedback #43(TRUE) -> (w781:bool)
            n541 = Not(x=w781) -> (.not. x?=w780:bool)
            n542 = feedback-in #43(w780) -> ()
            n543 = feedback #44(i16 0) -> (w794:i16)
            n544 = Subtract(x=w794, y=w792) -> (x-y=w793:i16)
            "DIO Relative phase" <- w793
            n545 = feedback-in #44(w793) -> ()
            n546 = Add(x=w799, y=w792) -> (x+y=w798:u32)
            n547 = Build Array "BD 1 nu Stack"(w825, w824, w823, w822, w821, w820) -> (w819:u8[])
            n548 = Not Equal?(x=w759, y=u8 3) -> (x != y?=w768:bool)
            n549 = case "Store in RF board F1 or F2" shown="True" w780 {
              tunnel: [w991 w995] -> w810
              tunnel: [u8 10 u8 4] -> w811
              tunnel: "Swap F1 and F2" -> [w992 w995]
              tunnel: "BD 2 Frequency 1" -> [_ w994]
              tunnel: "BD 2 Frequency 2" -> [w990 _]
              tunnel: [w990 w994] -> w776
              frame False {
                # "for RF synth controls\ngreen: F1/F2 stay same"
                # "F2 address (hex)"
                n550 = Not(x=w992) -> (.not. x?=w991:bool)
              }
              frame True {
                # "low chooses F1"
                # "F1 address (hex)"
              }
            }
            n551 = Select(t=w776, s="RF synth bd controls green", f=w775) -> (s? t:f=w774:u64)
            n552 = Split Number(x=w774) -> (hi(x)=w830:u32, lo(x)=w829:u32)
            n553 = Split Number(x=w830) -> (lo(x)=w828:u16)  [unwired: 1 out]
            n554 = Split Number(x=w829) -> (hi(x)=w827:u16, lo(x)=w826:u16)
            n555 = Split Number(x=w828) -> (hi(x)=w818:u8, lo(x)=w817:u8)
            n556 = Split Number(x=w827) -> (hi(x)=w816:u8, lo(x)=w815:u8)
            n557 = Split Number(x=w826) -> (hi(x)=w814:u8, lo(x)=w813:u8)
            n558 = feedback #45(u16 0 ("BD 2 Amplitude 3")) -> (w765:u16)
            n559 = Select(t=w765, s=w768, f=w767) -> (s? t:f=w766:u16)
            n560 = feedback-in #45(w766) -> ()
            n561 = And(x=w768, y=w771) -> (x .and. y?=w770:bool)
            n562 = Build Array "BD 2 nu Stack"(w818, w817, w816, w815, w814, w813) -> (w812:u8[])
            n563 = Select(t=w765, s=w770, f=w767) -> (s? t:f=w748:u16)
            n564 = flat-sequence "Update trap RF synth board settings to be used for the upcoming trap cycle." {
              tunnel: w812 -> [w939]
              tunnel: w819 -> [w940]
              tunnel: [w940] -> w763
              tunnel: [w939] -> w762
              tunnel: w811 -> [w941]
              tunnel: w763 -> [w943]
              tunnel: w762 -> [w942]
              tunnel: w750 -> [w954]
              tunnel: w752 -> [w953]
              tunnel: w751 -> [w952]
              frame #0 {
                # "To possibly delay\nthese writes to very\nend of loop (for x and\ny phase adjust)"
                n565 = call "Wait8"("Count(Ticks)"="Next trap write delay (ticks)") -> ()  [unwired: 1 out]
              }
              frame #1 {
                # "Next trap RF frequency:\n\nWrite next trap cycle frequency to buffer."
                n566 = for {
                  tunnel: w943 -> [w949] mode=indexing
                  tunnel: w942 -> [w948] mode=indexing
                  tunnel: w941 -> [w946]
                  i -> [w947]
                  n567 = To Unsigned Byte Integer(number=w947) -> (unsigned 8bit integer=w944:u8)
                  n568 = Add(x=w946, y=w944) -> (x+y=w945:u8)
                  n569 = call "write to RF synth bd.vi"("Address Byte"=w945, "BD 2 Byte"=w948, "BD 1 Byte"=w949) -> ()
                }
              }
              frame #2 {
                w950 = TRUE ("Connector1/DIO15")
                # "Send udclk high\n(BD 1 and 2) to make the new frequency active in F1 or F2 word. But it won't actually be the used frequency until FSK switches to it (begining of next cycle)."
                n570 = xnode "FPGA I/O Node"("Connector1/DIO30"=w950, "Connector1/DIO29"=w950) -> ()  [unwired: 2 in, 2 out]
              }
              frame #3 {
                w951 = FALSE ("Connector1/DIO15")
                n571 = xnode "FPGA I/O Node"("Connector1/DIO30"=w951, "Connector1/DIO29"=w951) -> ()  [unwired: 2 in, 2 out]
              }
              frame #4 {
                # "Next trap RF phase offset:\n\nSet the next trap cycle amplitude to the buffer. Won't become active until udclk is set high at proper time at the begining of the next cycle."
                n572 = case shown="True" w954 {
                  tunnel: w953 -> [_ w955]
                  tunnel: w952 -> [_ w956]
                  frame False {
                  }
                  frame True {
                    # "phase 1 address start"
                    n573 = for {
                      tunnel: w955 -> [w963] mode=indexing
                      tunnel: w956 -> [w962] mode=indexing
                      tunnel: u8 0 -> [w960]
                      i -> [w961]
                      n574 = To Unsigned Byte Integer(number=w961) -> (unsigned 8bit integer=w958:u8)
                      n575 = Add(x=w960, y=w958) -> (x+y=w959:u8)
                      n576 = call "write to RF synth bd.vi"("Address Byte"=w959, "BD 2 Byte"=w962, "BD 1 Byte"=w963) -> ()
                    }
                  }
                }
              }
              frame #5 {
                # "Prep to reset RF phase to zero at start of next cycle. Only reset BD 1. Do nothing to BD 2. This puts the settings in the buffer. A udclk high will make both this phase reset and possibly a new phase offset setting active."
                n577 = case shown="True" "RF phase reset before cycles" {
                  frame False {
                  }
                  frame True {
                    w966 = u8 66  # BD 1 reset
                    n578 = call "write to RF synth bd.vi"("Address Byte"=u8 31, "BD 2 Byte"=u8 2, "BD 1 Byte"=w966) -> ()
                  }
                }
              }
              frame #6 {
                # "Address"
                # "Data BD 2"
                # "Data BD 1"
                # "If phase reset wasn't chosen previously, these actions will have no affect. For both BD's, data should be binary 10, and address should be hex 1F (bin 01 1111)"
                # "This sets up the digital communication lines to restart phase accumulation (start RF running agin). It cancels out the possible phase reset. Just need to set WR DIO low then udclk DIOhigh  to make this happen. Doing this here early (and not using the usual board write function) speeds things up.\n\nRestarts RF (BD 1 only, BD2 never stopped in first place)."
                n579 = xnode "FPGA I/O Node"("Connector1/DIO0"=FALSE, "Connector1/DIO1"=FALSE, "Connector1/DIO2"=FALSE, "Connector1/DIO3"=FALSE, "Connector1/DIO4"=FALSE, "Connector1/DIO5"=FALSE, "Connector1/DIO6"=TRUE, "Connector1/DIO7"=FALSE, "Connector1/DIO8"=FALSE, "Connector1/DIO9"=TRUE, "Connector1/DIO10"=TRUE, "Connector1/DIO11"=TRUE, "Connector1/DIO12"=TRUE, "Connector1/DIO13"=TRUE, "Connector1/DIO20"=FALSE, "Connector1/DIO21"=FALSE, "Connector1/DIO22"=FALSE, "Connector1/DIO23"=FALSE, "Connector1/DIO24"=FALSE, "Connector1/DIO25"=FALSE, "Connector1/DIO26"=TRUE, "Connector1/DIO27"=FALSE) -> ()  [unwired: 22 in, 22 out]
              }
            }
            n580 = feedback #46(fxp<+,8,8> 0.0) -> (w745:fxp<+,8,8>)
            n581 = Increment(x=w745) -> (x+1=w743:fxp<+,8,8>)
            n582 = feedback-in #46(w743) -> ()
            n583 = case "Trap RF phase offset control methods" shown="3" "Phase offset method" {
              tunnel: [fxp<+,14,14> 0.0 ("Phase BD 1") w889 w904 w933] -> w753
              tunnel: "Phase Trap 1" -> [_ w890 w905 _]
              tunnel: w759 -> [_ w891 w906 w934]
              tunnel: [FALSE TRUE TRUE TRUE] -> w750
              tunnel: "Phase Trap 2" -> [_ w887 w902 _]
              tunnel: w743 -> [_ _ w901 _]
              frame 0, Default {
              }
              frame 1 {
                # "Constant increment of phase offset with each trap cycle. This results in a constant phase difference between trap cycles. \nOnly for traps 1 and 2 (set phase offset to zero for set three)."
                n584 = case shown="1, Default" w891 {
                  tunnel: w890 -> [_ _ w897]
                  tunnel: [w893 fxp<+,14,14> 0.0 w898] -> w889
                  tunnel: w887 -> [w892 _ _]
                  frame 2 {
                    n585 = feedback #47(fxp<+,14,14> 0.0) -> (w895:fxp<+,14,14>)
                    n586 = Add(x=w892, y=w895) -> (x+y=w893:fxp<+,14,14>)
                    n587 = feedback-in #47(w893) -> ()
                  }
                  frame 3 {
                  }
                  frame 1, Default {
                    n588 = feedback #48(fxp<+,14,14> 0.0) -> (w900:fxp<+,14,14>)
                    n589 = Add(x=w897, y=w900) -> (x+y=w898:fxp<+,14,14>)
                    n590 = feedback-in #48(w898) -> ()
                  }
                }
              }
              frame 2 {
                # "Changing increment of phase offset with each trap cycle. This results in a constant change in phase difference between trap cycles. \nOnly for traps 1 and 2 (set phase offset to zero for set three)."
                n591 = case shown="2" w906 {
                  tunnel: w905 -> [_ _ w916]
                  tunnel: [w907 fxp<+,14,14> 0.0 w914] -> w904
                  tunnel: w902 -> [w909 _ _]
                  tunnel: w901 -> [w910 _ w917]
                  frame 2 {
                    n592 = Multiply(x=w909, y=w910) -> (x*y=w908:fxp<+,16,16>)
                    n593 = feedback #49(fxp<+,14,14> 0.0) -> (w912:fxp<+,14,14>)
                    n594 = Add(x=w908, y=w912) -> (x+y=w907:fxp<+,14,14>)
                    n595 = feedback-in #49(w907) -> ()
                  }
                  frame 3 {
                  }
                  frame 1, Default {
                    n596 = Multiply(x=w916, y=w917) -> (x*y=w915:fxp<+,16,16>)
                    n597 = feedback #50(fxp<+,14,14> 0.0) -> (w919:fxp<+,14,14>)
                    n598 = Add(x=w915, y=w919) -> (x+y=w914:fxp<+,14,14>)
                    n599 = feedback-in #50(w914) -> ()
                  }
                }
              }
              frame 3 {
                w926 = u32 1013904223  # LCG constant C (add)
                w928 = fxp<+,21,21> 1664525.0  # LCG constant A (multiply)
                # "Set a random phase offset. Random number generated using the LCG method. Constants and method taken from NI white noise generator code (method is general though)."
                # "shift to 14 significant bits"
                n600 = feedback #51(u32 4294967295 ("seed")) -> (w923:u32)
                n601 = Multiply(x=w923, y=w928) -> (x*y=w927:u32)
                n602 = Split Number(x=w923) -> (hi(x)=w929:u16)  [unwired: 1 out]
                n603 = To Unsigned Word Integer(number=w929) -> (unsigned 16bit integer=w921:u16)
                n604 = Add(x=w927, y=w926) -> (x+y=w925:fxp<+,32,32>)
                n605 = To Unsigned Long Integer(number=w925) -> (unsigned 32bit integer=w922:u32)
                n606 = feedback-in #51(w922) -> ()
                n607 = Scale By Power Of 2(n=i8 -2 ("Uniform scale factor"), x=w921) -> (x*2^n=w930:u16)
                n608 = To Fixed-Point(number=w930) -> (fixed-point=w920:fxp<+,14,14>)  [unwired: 1 in]
                "Random phase generated" <- w920
                n609 = case shown="1, Default" w934 {
                  tunnel: [w935 fxp<+,14,14> 0.0 w937] -> w933
                  tunnel: w920 -> [w935 _ w937]
                  frame 2 {
                  }
                  frame 3 {
                  }
                  frame 1, Default {
                  }
                }
              }
            }
            n610 = To Unsigned Word Integer(number=w753) -> (unsigned 16bit integer=w758:u16)
            n611 = Split Number(x=w758) -> (hi(x)=w756:u8, lo(x)=w757:u8)
            n612 = Split Number(x=u16 0) -> (hi(x)=w754:u8, lo(x)=w755:u8)
            n613 = Build Array ("BD 1 A Stack")(w756, w757) -> (w752:u8[])
            n614 = Build Array ("BD 1 A Stack")(w754, w755) -> (w751:u8[])
          }
        }
      }
    }
  }
  n615 = while "532 nm green fluorescent laser interlacing (DO to IA 532 nm AOM ME amp)." {
    shift-right: [w1299] -> _
    shift-left: w2 -> [w1304]
    shift-right: [w1298] -> _
    shift-left: w5 -> [w1296]
    stop <- FALSE stop-if-true
    n616 = flat-sequence {
      tunnel: w1304 -> [w1307]
      tunnel: [w1306] -> w1302
      tunnel: [w1307] -> w1300
      tunnel: [w1308] -> w1297
      tunnel: w1296 -> [w1308]
      tunnel: [w1311] -> w1303
      tunnel: w1302 -> [w1311]
      tunnel: [w1310] -> w1301
      tunnel: w1300 -> [w1310]
      tunnel: w1297 -> [w1309]
      tunnel: [w1320] -> w1299
      tunnel: w1303 -> [w1340]
      tunnel: w1301 -> [w1337]
      tunnel: [w1329] -> w1298
      frame #0 {
        n617 = call "Loop Timer9"("Count(Ticks)"=w1307) -> ("Tick Count(Ticks)"=w1306:u32)
      }
      frame #1 {
        # "Then to PRL 440 amp\nOR to RF synth board FSK in"
        n618 = xnode "FPGA I/O Node"("Connector1/DIO37"=w1309, "Connector1/DIO38"=w1309, "Connector1/DIO39"=w1309, "Connector1/DIO26"=w1309, "Connector1/DIO32"=w1309) -> ()  [unwired: 5 in, 5 out]
      }
      frame #2 {
        n619 = feedback-in #52(w1340) -> ()
        n620 = feedback #52(w1340) -> (w1339:u32)
        n621 = Subtract(x=w1340, y=w1339) -> (x-y=w1338:u32)
        n622 = Subtract(x=w1338, y=w1337) -> (x-y=w1313:u32)
        n623 = Number To Boolean Array(number=w1313) -> (Boolean array=w1314:bool[])
        n624 = Or Array Elements(Boolean array=w1314) -> (logical OR=w1312:bool)
        n625 = Boolean To (0,1)(Boolean="+ phase (GI)") -> (0, 1=w1325:i16)
        n626 = Multiply(x=w1325, y="Phase count adjustment (GI)") -> (x*y=w1322:i16)
        n627 = Boolean To (0,1)(Boolean=w1312) -> (0, 1=w1319:i16)
        n628 = To Unsigned Byte Integer(number=w1319) -> (unsigned 8bit integer=w1316:u8)
        n629 = feedback #53(i16 0) -> (w1323:i16)
        n630 = feedback #54(u8 0) -> (w1317:u8)
        n631 = Add(x=w1316, y=w1317) -> (x+y=w1315:u8)
        "GI Late Counter" <- w1315
        n632 = feedback-in #54(w1315) -> ()
        n633 = Subtract(x=w1323, y=w1322) -> (x-y=w1321:i16)
        "GI Relative phase" <- w1321
        n634 = feedback-in #53(w1321) -> ()
        n635 = feedback #55(TRUE) -> (w1332:bool)
        n636 = case shown="0, Default" "Operating Mode" {
          tunnel: [TRUE FALSE w1346] -> w1329
          tunnel: w1332 -> [_ _ w1343]
          frame 0, Default {
          }
          frame 1 {
          }
          frame 2 {
            n637 = Not(x=w1343) -> (.not. x?=w1345:bool)
            n638 = Select(t=w1345, s="Invert GI", f=w1343) -> (s? t:f=w1346:bool)
          }
        }
        n639 = Not(x=w1332) -> (.not. x?=w1328:bool)
        n640 = Select(t="Green interlace ON count", s=w1328, f="Green interlace OFF count") -> (s? t:f=w1334:u16)
        n641 = Subtract(x=w1334, y=w1313) -> (x-y=w1326:u32)
        n642 = Add(x=w1326, y=w1322) -> (x+y=w1320:u32)
        n643 = feedback-in #55(w1328) -> ()
      }
    }
  }
  n644 = while "Green excitation laser feedback measurement" {
    shift-right: [w1347] -> _
    shift-left: w2 -> [w1352]
    stop <- FALSE stop-if-true
    n645 = flat-sequence {
      tunnel: w1352 -> [w1354]
      tunnel: [w1355] -> w1350
      tunnel: [w1354] -> w1348
      tunnel: [w1362] -> w1351
      tunnel: w1350 -> [w1362]
      tunnel: [w1361] -> w1349
      tunnel: w1348 -> [w1361]
      tunnel: [w1374] -> w1347
      tunnel: w1351 -> [w1385]
      tunnel: w1349 -> [w1382]
      frame #0 {
        n646 = call "Loop Timer6"("Count(Ticks)"=w1354) -> ("Tick Count(Ticks)"=w1355:u32)
      }
      frame #1 {
        n647 = xnode "FPGA I/O Node"("Connector1/DIO35"=TRUE) -> ("Chassis2/Mod2/AI0"=w1360:i16, "Chassis2/Mod2/AI1"=w1359:i16, "Chassis2/Mod2/AI2"=w1356:i16)  [unwired: 4 in, 4 out]
        "Green FB Sum" <- w1356
        n648 = Bundle("Chassis2/Mod2/AI0"=w1360, "Chassis2/Mod2/AI1"=w1359, "Chassis2/Mod2/AI2"=w1356) -> (→"Green FB Signals":T10)  [unwired: 1 out]
      }
      frame #2 {
        n649 = feedback-in #56(w1385) -> ()
        n650 = feedback #56(w1385) -> (w1384:u32)
        n651 = Subtract(x=w1385, y=w1384) -> (x-y=w1383:u32)
        n652 = xnode "FPGA I/O Node"("Connector1/DIO35"=FALSE) -> ()  [unwired: 1 in, 1 out]
        n653 = Subtract(x=w1383, y=w1382) -> (x-y=w1364:u32)
        n654 = Subtract(x="Green FB Count", y=w1364) -> (x-y=w1378:u32)
        n655 = Number To Boolean Array(number=w1364) -> (Boolean array=w1365:bool[])
        n656 = Or Array Elements(Boolean array=w1365) -> (logical OR=w1363:bool)
        "Green FB Late?" <- w1363
        n657 = Boolean To (0,1)(Boolean="+ phase (Green FB)") -> (0, 1=w1376:i16)
        n658 = Boolean To (0,1)(Boolean=w1363) -> (0, 1=w1370:i16)
        n659 = Multiply(x=w1376, y="Phase count adjustment (Green FB)") -> (x*y=w1371:i16)
        n660 = Add(x=w1378, y=w1371) -> (x+y=w1374:u32)
        n661 = To Unsigned Word Integer(number=w1370) -> (unsigned 16bit integer=w1367:u16)
        n662 = feedback #57(i16 0) -> (w1373:i16)
        n663 = Subtract(x=w1373, y=w1371) -> (x-y=w1372:i16)
        "Green FB Relative Phase" <- w1372
        n664 = feedback-in #57(w1372) -> ()
        n665 = feedback #58(u16 0) -> (w1368:u16)
        n666 = Add(x=w1367, y=w1368) -> (x+y=w1366:u16)
        "Green Late Counter" <- w1366
        n667 = feedback-in #58(w1366) -> ()
      }
    }
  }
  n668 = while "Control APD data integration - stream to host" {
    shift-right: [w1388] -> _
    shift-left: w7 -> [w1393]
    stop <- FALSE stop-if-true
    n669 = flat-sequence {
      tunnel: w1393 -> [w1395]
      tunnel: [w1396] -> w1391
      tunnel: [w1395] -> w1389
      tunnel: [w1404] -> w1392
      tunnel: w1391 -> [w1404]
      tunnel: [w1403] -> w1390
      tunnel: w1389 -> [w1403]
      tunnel: [w1402] -> w1387
      tunnel: [w1401] -> w1386
      tunnel: [w1438] -> w1388
      tunnel: w1392 -> [w1450]
      tunnel: w1390 -> [w1447]
      tunnel: w1387 -> [w1431]
      tunnel: w1386 -> [w1430]
      frame #0 {
        n670 = call "Loop Timer4"("Count(Ticks)"=w1395) -> ("Tick Count(Ticks)"=w1396:u32)
      }
      frame #1 {
        n671 = flat-sequence {
          tunnel: [w1406] -> w1400
          tunnel: w1400 -> [w1408]
          tunnel: [w1410] -> w1399
          tunnel: [w1409] -> w1398
          tunnel: [w1408] -> w1397
          tunnel: [w1416] -> w1401
          tunnel: [w1417] -> w1402
          tunnel: w1399 -> [w1417]
          tunnel: w1398 -> [w1416]
          tunnel: w1397 -> [w1415]
          frame #0 {
            # "use two separate variable so each APD won't\nhave to wait to read"
            n672 = feedback #59(FALSE) -> (w1405:bool)
            "APD1 out state" <- w1405
            "APD2 out state" <- w1405
            n673 = Not(x=w1405) -> (.not. x?=w1406:bool)
            n674 = feedback-in #59(w1406) -> ()
            n675 = xnode "FPGA I/O Node"("Connector0/DIO5"=w1405) -> ()  [unwired: 1 in, 1 out]
          }
          frame #1 {
            n676 = local read "APD 1 Counts 1"() -> (w1414:u32)
            n677 = local read "APD 1 Counts 0"() -> (w1413:u32)
            n678 = local read "APD 2 Counts 1"() -> (w1412:u32)
            n679 = local read "APD 2 Counts 0"() -> (w1411:u32)
            n680 = Select(t=w1414, s=w1408, f=w1413) -> (s? t:f=w1410:u32)
            n681 = Select(t=w1412, s=w1408, f=w1411) -> (s? t:f=w1409:u32)
          }
          frame #2 {
            n682 = case shown="True" w1415 {
              frame False {
                w1418 = u32 0 ("APD 1 Counts 0")
                n683 = local write "APD 1 Counts 0"(w1418) -> ()
                n684 = local write "APD 2 Counts 0"(w1418) -> ()
              }
              frame True {
                w1419 = u32 0 ("APD 1 Counts 1")
                n685 = local write "APD 1 Counts 1"(w1419) -> ()
                n686 = local write "APD 2 Counts 1"(w1419) -> ()
              }
            }
          }
        }
      }
      frame #2 {
        n687 = feedback-in #60(w1450) -> ()
        n688 = feedback #60(w1450) -> (w1449:u32)
        n689 = Subtract(x=w1450, y=w1449) -> (x-y=w1448:u32)
        n690 = Subtract(x=w1448, y=w1447) -> (x-y=w1423:u32)
        n691 = case shown="True" "APD to FIFO" {
          tunnel: w1431 -> [_ w1453]
          tunnel: w1430 -> [_ w1451]
          frame False {
          }
          frame True {
            n692 = flat-sequence {
              tunnel: 0 ("Timeout") -> [w1455]
              tunnel: w1453 -> [w1456]
              tunnel: [w1455] -> w1452
              tunnel: w1452 -> [w1458]
              tunnel: w1451 -> [w1457]
              frame #0 {
                n693 = xnode ("FIFO Write")("Element"=w1456, "Timeout"=w1455) -> ()  [unwired: 1 in, 2 out]
              }
              frame #1 {
                n694 = xnode ("FIFO Write")("Element"=w1457, "Timeout"=w1458) -> ()  [unwired: 1 in, 2 out]
              }
            }
          }
        }
        n695 = Subtract(x="APD Acq Rate Count", y=w1423) -> (x-y=w1439:u32)
        n696 = Number To Boolean Array(number=w1423) -> (Boolean array=w1424:bool[])
        n697 = Or Array Elements(Boolean array=w1424) -> (logical OR=w1422:bool)
        "APD Acq Late?" <- w1422
        n698 = Boolean To (0,1)(Boolean=w1422) -> (0, 1=w1429:i16)
        n699 = To Unsigned Word Integer(number=w1429) -> (unsigned 16bit integer=w1426:u16)
        n700 = Boolean To (0,1)(Boolean="+ phase (APD Acq)") -> (0, 1=w1435:i16)
        n701 = feedback #61(u16 0) -> (w1427:u16)
        n702 = Add(x=w1426, y=w1427) -> (x+y=w1425:u16)
        "APD Acq Late Counter" <- w1425
        n703 = feedback-in #61(w1425) -> ()
        n704 = Multiply(x=w1435, y="Phase Count Adjustment (APD Acq)") -> (x*y=w1432:i16)
        n705 = Add(x=w1439, y=w1432) -> (x+y=w1438:u32)
        n706 = feedback #62(i16 0) -> (w1437:i16)
        n707 = Subtract(x=w1437, y=w1432) -> (x-y=w1434:i16)
        "APD Acq Relative Phase" <- w1434
        n708 = feedback-in #62(w1434) -> ()
        n709 = To Word Integer(number=w1431) -> (16bit integer=w1440:i16)
        n710 = To Word Integer(number=w1430) -> (16bit integer=w1441:i16)
        n711 = Multiply(x="APD 1 AO scale factor", y=w1440) -> (x*y=w1421:i16)
        n712 = Multiply(x="APD 2 AO scale factor", y=w1441) -> (x*y=w1420:i16)
        n713 = xnode "FPGA I/O Node"("Connector0/AO6"=w1421, "Connector0/AO7"=w1420) -> ()  [unwired: 2 in, 2 out]
      }
    }
  }
  n714 = disable-structure shown="Disabled" {
    disable-tunnel: w2 -> [w1461 _]
    disable-tunnel: w5 -> [w1460 _]
    frame Disabled {
      n715 = while "633 nm red  fluorescent laser interlacing (DO to IA 633 nm AOM ME amp)." {
        shift-right: [w1582] -> _
        shift-left: w1461 -> [w1587]
        shift-right: [w1581] -> _
        shift-left: w1460 -> [w1579]
        stop <- FALSE stop-if-true
        n716 = flat-sequence {
          tunnel: w1587 -> [w1590]
          tunnel: [w1589] -> w1585
          tunnel: [w1590] -> w1583
          tunnel: [w1591] -> w1580
          tunnel: w1579 -> [w1591]
          tunnel: [w1594] -> w1586
          tunnel: w1585 -> [w1594]
          tunnel: [w1593] -> w1584
          tunnel: w1583 -> [w1593]
          tunnel: w1580 -> [w1592]
          tunnel: [w1603] -> w1582
          tunnel: w1586 -> [w1623]
          tunnel: w1584 -> [w1620]
          tunnel: [w1612] -> w1581
          frame #0 {
            n717 = call "Loop Timer8"("Count(Ticks)"=w1590) -> ("Tick Count(Ticks)"=w1589:u32)
          }
          frame #1 {
            # "Then to PRL 440 amp"
            n718 = xnode "FPGA I/O Node"("Connector1/DIO32"=w1592) -> ()  [unwired: 1 in, 1 out]
          }
          frame #2 {
            n719 = feedback-in #63(w1623) -> ()
            n720 = feedback #63(w1623) -> (w1622:u32)
            n721 = Subtract(x=w1623, y=w1622) -> (x-y=w1621:u32)
            n722 = Subtract(x=w1621, y=w1620) -> (x-y=w1596:u32)
            n723 = Number To Boolean Array(number=w1596) -> (Boolean array=w1597:bool[])
            n724 = Or Array Elements(Boolean array=w1597) -> (logical OR=w1595:bool)
            n725 = Boolean To (0,1)(Boolean="+ phase (RI)") -> (0, 1=w1608:i16)
            n726 = Multiply(x=w1608, y="Phase count adjustment (RI)") -> (x*y=w1605:i16)
            n727 = Boolean To (0,1)(Boolean=w1595) -> (0, 1=w1602:i16)
            n728 = To Unsigned Byte Integer(number=w1602) -> (unsigned 8bit integer=w1599:u8)
            n729 = feedback #64(i16 0) -> (w1606:i16)
            n730 = feedback #65(u8 0) -> (w1600:u8)
            n731 = Add(x=w1599, y=w1600) -> (x+y=w1598:u8)
            "RI Late Counter" <- w1598
            n732 = feedback-in #65(w1598) -> ()
            n733 = Subtract(x=w1606, y=w1605) -> (x-y=w1604:i16)
            "RI Relative phase" <- w1604
            n734 = feedback-in #64(w1604) -> ()
            n735 = feedback #66(TRUE) -> (w1615:bool)
            n736 = case shown="2" "Red Laser Operating Mode" {
              tunnel: [TRUE FALSE w1629] -> w1612
              tunnel: w1615 -> [_ _ w1626]
              frame 0, Default {
              }
              frame 1 {
              }
              frame 2 {
                n737 = Not(x=w1626) -> (.not. x?=w1628:bool)
                n738 = Select(t=w1628, s="Invert RI", f=w1626) -> (s? t:f=w1629:bool)
              }
            }
            n739 = Not(x=w1615) -> (.not. x?=w1611:bool)
            n740 = Select(t="Red interlace ON count", s=w1611, f="Red interlace OFF count") -> (s? t:f=w1617:u16)
            n741 = Subtract(x=w1617, y=w1596) -> (x-y=w1609:u32)
            n742 = Add(x=w1609, y=w1605) -> (x+y=w1603:u32)
            n743 = feedback-in #66(w1611) -> ()
          }
        }
      }
      n744 = while "473 nm blue  fluorescent laser interlacing (DO to blue laser digital control input)." {
        shift-right: [w1478] -> _
        shift-left: w1461 -> [w1481]
        shift-right: [w1477] -> _
        shift-left: w1460 -> [w1475]
        shift-right: [w1470] -> _
        shift-left: _ -> [w1469]
        shift-right: [w1462] -> _
        shift-left: u16 0 -> [w1465]
        stop <- FALSE stop-if-true
        n745 = flat-sequence {
          tunnel: w1481 -> [w1484]
          tunnel: [w1483] -> w1480
          tunnel: [w1484] -> w1479
          tunnel: [w1487] -> w1476
          tunnel: w1475 -> [w1487]
          tunnel: w1469 -> [w1486]
          tunnel: [w1486] -> w1468
          tunnel: [w1485] -> w1466
          tunnel: w1465 -> [w1485]
          tunnel: [w1492] -> w1474
          tunnel: w1480 -> [w1492]
          tunnel: [w1491] -> w1473
          tunnel: w1479 -> [w1491]
          tunnel: w1476 -> [w1490]
          tunnel: w1468 -> [w1489]
          tunnel: [w1489] -> w1467
          tunnel: w1466 -> [w1488]
          tunnel: [w1488] -> w1464
          tunnel: [w1497] -> w1472
          tunnel: [w1496] -> w1471
          tunnel: w1473 -> [w1496]
          tunnel: w1474 -> [w1497]
          tunnel: w1467 -> [w1495]
          tunnel: w1464 -> [w1494]
          tunnel: [w1493] -> w1463
          tunnel: [w1554] -> w1478
          tunnel: w1472 -> [w1572]
          tunnel: w1471 -> [w1569]
          tunnel: [w1542] -> w1477
          tunnel: [w1540] -> w1470
          tunnel: w1463 -> [w1537]
          tunnel: [w1538] -> w1462
          frame #0 {
            n746 = call "Loop Timer7"("Count(Ticks)"=w1484) -> ("Tick Count(Ticks)"=w1483:u32)
          }
          frame #1 {
            n747 = xnode "FPGA I/O Node"("Connector1/DIO28"=w1490) -> ()  [unwired: 1 in, 1 out]
          }
          frame #2 {
            n748 = case shown="True" w1495 {
              tunnel: w1494 -> [w1498 w1500]
              tunnel: [w1498 w1499] -> w1493
              frame False {
              }
              frame True {
                n749 = flat-sequence {
                  tunnel: [w1506] -> w1503
                  tunnel: [w1505] -> w1502
                  tunnel: [w1504] -> w1501
                  tunnel: w1500 -> [w1504]
                  tunnel: w1503 -> [w1523]
                  tunnel: w1502 -> [w1520]
                  tunnel: w1501 -> [w1522]
                  tunnel: [w1521] -> w1499
                  frame #0 {
                    # "5 ns timing resolution"
                    n750 = node-c288() -> (w1509:T7)  [unwired: 1 in]
                    n751 = timed-loop {
                      timing: w1509 -> [_]
                      timing-out: [_] -> w1508
                      tunnel: "Lifetime timeout APD1" -> [w1515]
                      tunnel: [w1510] -> w1505
                      tunnel: [w1511] -> w1506
                      i -> [w1512]
                      stop <- w1514 stop-if-true
                      n752 = xnode "FPGA I/O Node"() -> ("Connector0/DIO5"=w1513:bool)  [unwired: 1 in, 1 out]
                      n753 = To Unsigned Word Integer(number=w1512) -> (unsigned 16bit integer=w1510:u16)
                      n754 = Equal?(x=w1515, y=w1510) -> (x = y?=w1511:bool)
                      n755 = Or(x=w1513, y=w1511) -> (x .or. y?=w1514:bool)
                    }
                    n756 = node-c288(w1508) -> ()
                  }
                  frame #1 {
                    n757 = Not(x=w1523) -> (.not. x?=w1524:bool)
                    n758 = case shown="True" w1524 {
                      tunnel: w1520 -> [_ w1526]
                      tunnel: w1522 -> [w1525 w1528]
                      tunnel: [w1525 w1527] -> w1521
                      frame False {
                        # "timed out, do nothing"
                      }
                      frame True {
                        # "photon detected,record time"
                        n759 = case shown="True" "Lifetime to FIFO" {
                          tunnel: w1526 -> [_ w1534]
                          tunnel: w1528 -> [w1530 w1532]
                          tunnel: [w1530 w1531] -> w1527
                          frame False {
                            # "don't record time\n(can't if doing force feedback)"
                          }
                          frame True {
                            # "number of events in fifo"
                            n760 = xnode ("FIFO Method Node")("Element"=w1534, "Timeout"=0) -> ()  [unwired: 1 in, 2 out]
                            n761 = Increment(x=w1532) -> (x+1=w1531:u16)
                          }
                        }
                        "lifetime (ticks)" <- w1526
                      }
                    }
                  }
                }
              }
            }
          }
          frame #3 {
            # "Reading fifo is tricky here since\nunknown # of events"
            # "For lifetime measurement:\nInterlacing and pulse falling"
            n762 = feedback-in #67(w1572) -> ()
            n763 = feedback #67(w1572) -> (w1571:u32)
            n764 = Subtract(x=w1572, y=w1571) -> (x-y=w1570:u32)
            n765 = Subtract(x=w1570, y=w1569) -> (x-y=w1547:u32)
            n766 = Number To Boolean Array(number=w1547) -> (Boolean array=w1548:bool[])
            n767 = Or Array Elements(Boolean array=w1548) -> (logical OR=w1546:bool)
            n768 = Boolean To (0,1)(Boolean="+ phase (BI D)") -> (0, 1=w1559:i16)
            n769 = Multiply(x=w1559, y="Phase count adjustment (BI D)") -> (x*y=w1556:i16)
            n770 = Boolean To (0,1)(Boolean=w1546) -> (0, 1=w1553:i16)
            n771 = To Unsigned Byte Integer(number=w1553) -> (unsigned 8bit integer=w1550:u8)
            n772 = feedback #68(i16 0) -> (w1557:i16)
            n773 = feedback #69(u8 0) -> (w1551:u8)
            n774 = Add(x=w1550, y=w1551) -> (x+y=w1549:u8)
            "Blue Late Counter (D)" <- w1549
            n775 = feedback-in #69(w1549) -> ()
            n776 = Subtract(x=w1557, y=w1556) -> (x-y=w1555:i16)
            "BI Relative phase (D)" <- w1555
            n777 = feedback-in #68(w1555) -> ()
            n778 = feedback #70(TRUE) -> (w1564:bool)
            n779 = case shown="2" "Blue Laser Operating Mode (D)" {
              tunnel: [TRUE FALSE w1578] -> w1542
              tunnel: w1564 -> [_ _ w1575]
              frame 0, Default {
              }
              frame 1 {
              }
              frame 2 {
                n780 = Not(x=w1575) -> (.not. x?=w1577:bool)
                n781 = Select(t=w1577, s="Invert BI (D)", f=w1575) -> (s? t:f=w1578:bool)
              }
            }
            n782 = Subtract(x=w1537, y="Lifetime events to read blue") -> (x-y=w1535:u16)
            n783 = Not(x=w1564) -> (.not. x?=w1562:bool)
            n784 = Select(t="Blue interlace ON count (D)", s=w1562, f="Blue interlace OFF count (D)") -> (s? t:f=w1566:u16)
            n785 = Subtract(x=w1566, y=w1547) -> (x-y=w1560:u32)
            n786 = Add(x=w1560, y=w1556) -> (x+y=w1554:u32)
            n787 = feedback-in #70(w1562) -> ()
            n788 = Select(t=w1535, s="Lifetime read blue fifo", f=w1537) -> (s? t:f=w1538:u16)
            "lifetime events in fifo" <- w1538
            n789 = Equal?(x="Blue Laser Operating Mode (D)", y=u8 2) -> (x = y?=w1543:bool)
            n790 = Not(x=w1542) -> (.not. x?=w1541:bool)
            n791 = And(x=w1541, y=w1543) -> (x .and. y?=w1540:bool)
          }
        }
      }
    }
    frame Enabled {
    }
  }
